vi "myRIO_BRig_RT_dataMTrig_main.vi"(0 "input_dataMTrig":u16[](array[numeric]), 2 "input_Solenoid_trig_L":bool, 3 "input_Solenoid_trig_R":bool, 4 "input_Audio_trig_L":bool, 5 "input_Audio_trig_R":bool, 7 "input_Laser_trig":bool) -> (13 "output_Laser":bool, 14 "output_dataMTrig":u16[](array[numeric]), 16 "output_Solenoid_L":bool, 17 "output_Solenoid_R":bool, 18 "output_Audio_L":bool, 19 "output_Audio_R":bool)   [LabVIEW 2014]
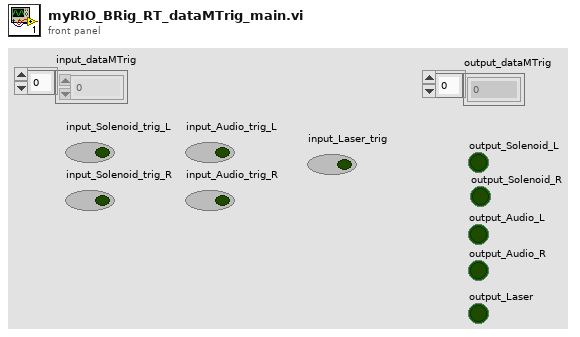
[diagram p1: front panel]
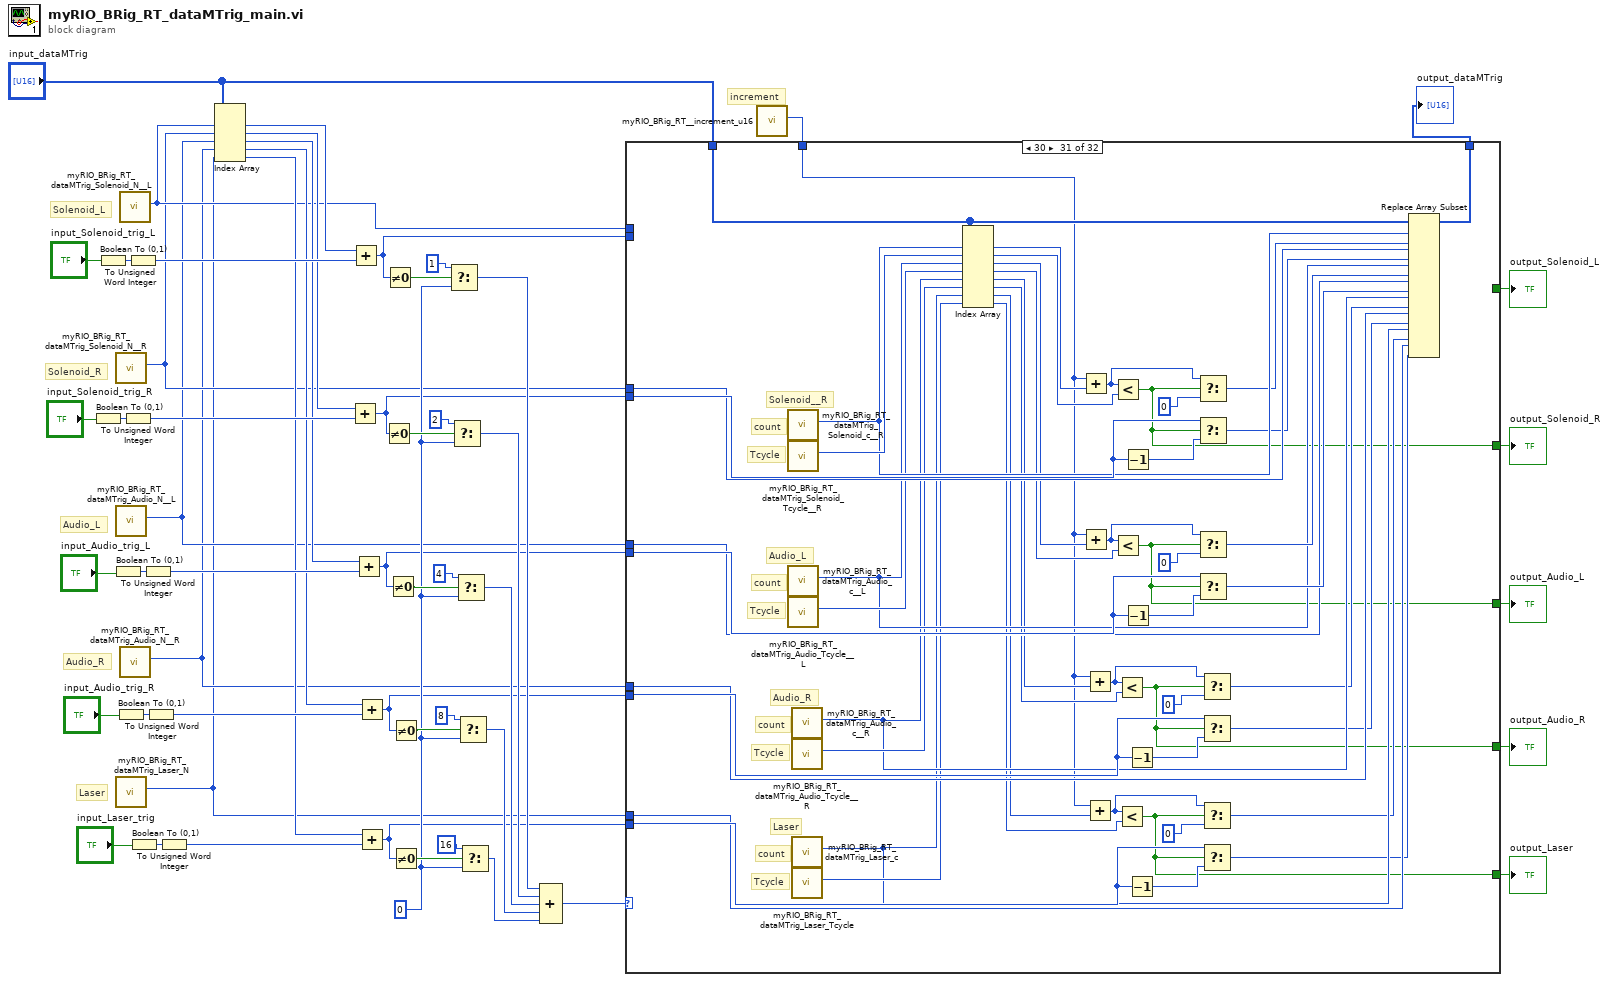
[diagram p0: block diagram]
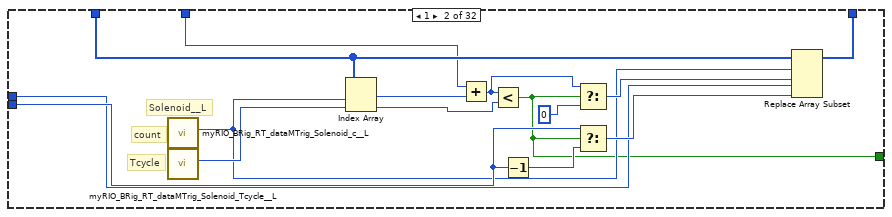
[diagram p3: hidden frame]
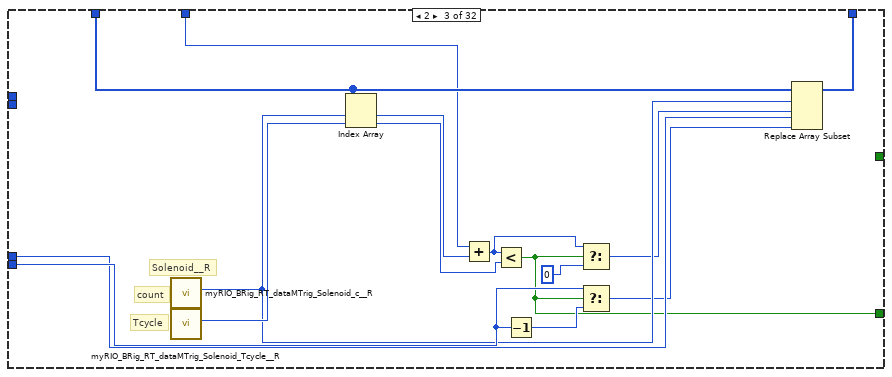
[diagram p4: hidden frame]
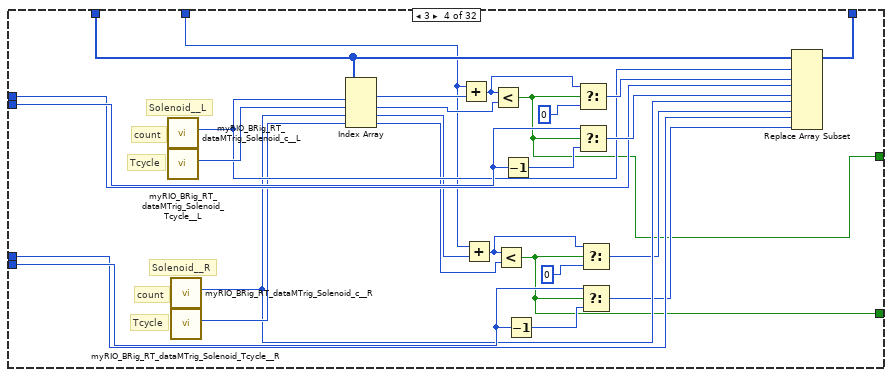
[diagram p5: hidden frame]
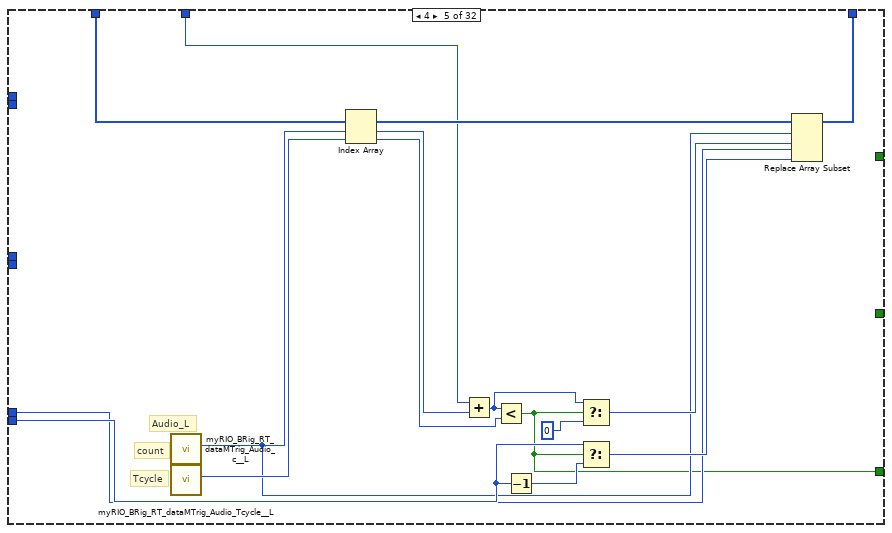
[diagram p6: hidden frame]
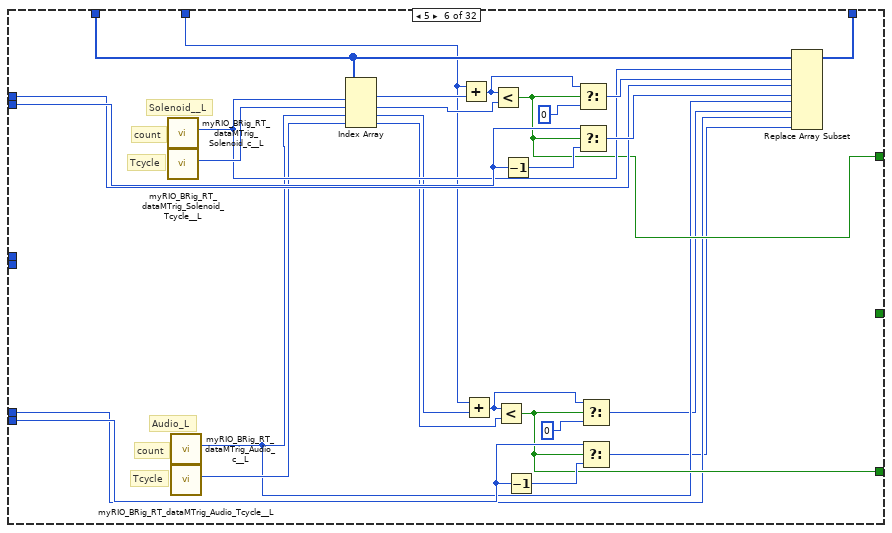
[diagram p7: hidden frame]
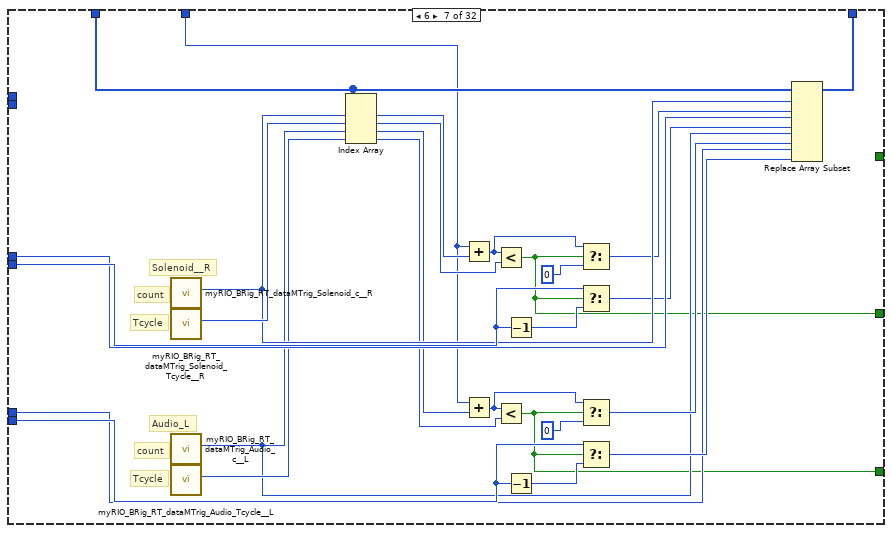
[diagram p8: hidden frame]
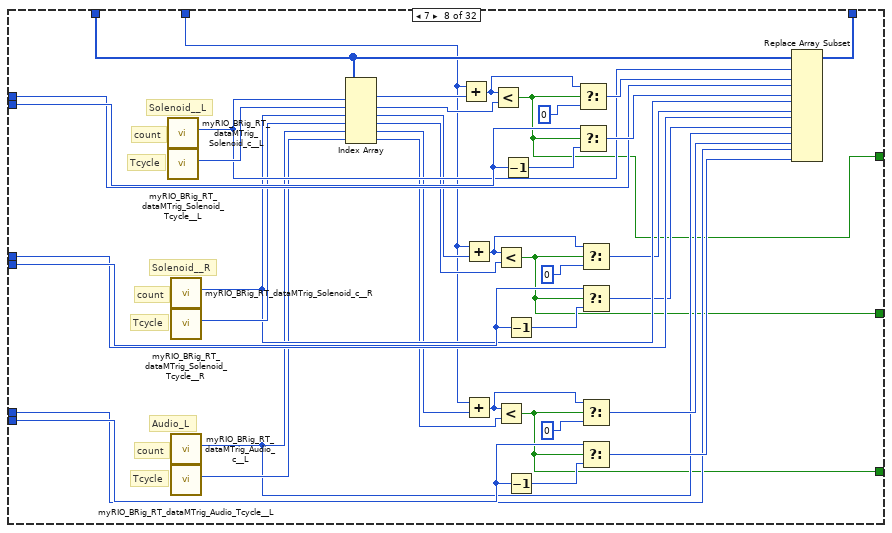
[diagram p9: hidden frame]
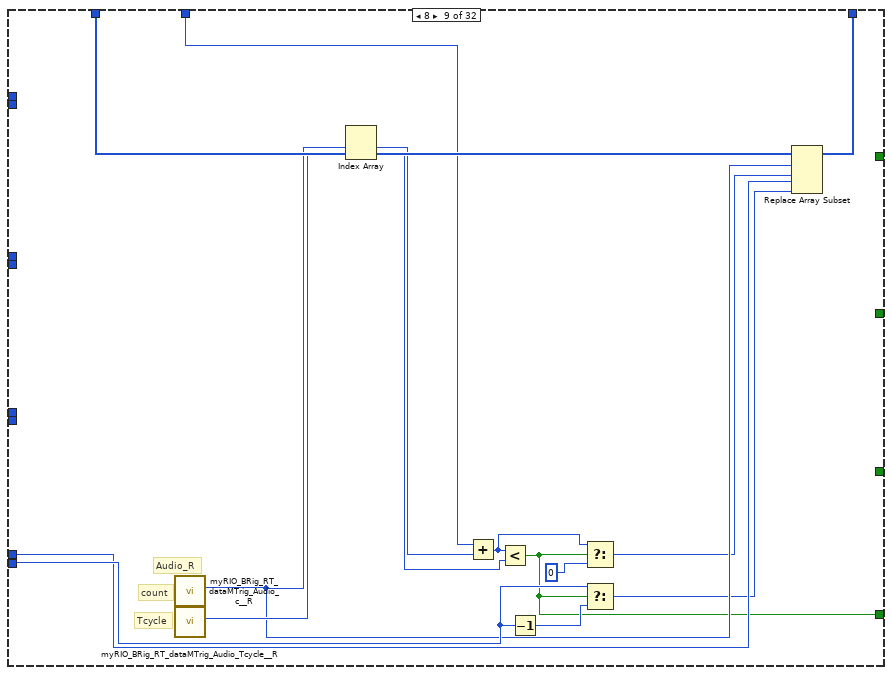
[diagram p10: hidden frame]
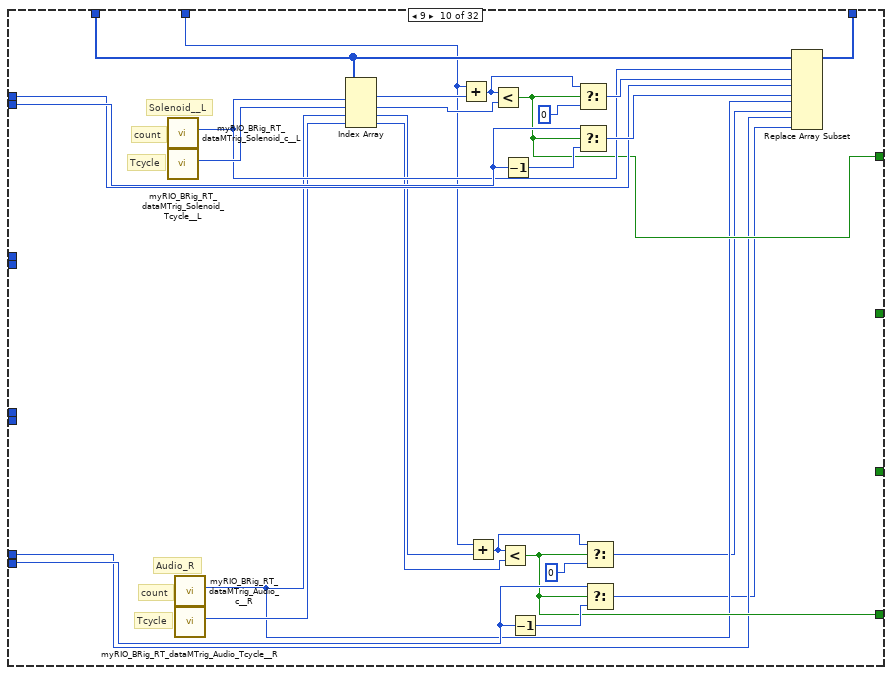
[diagram p11: hidden frame]
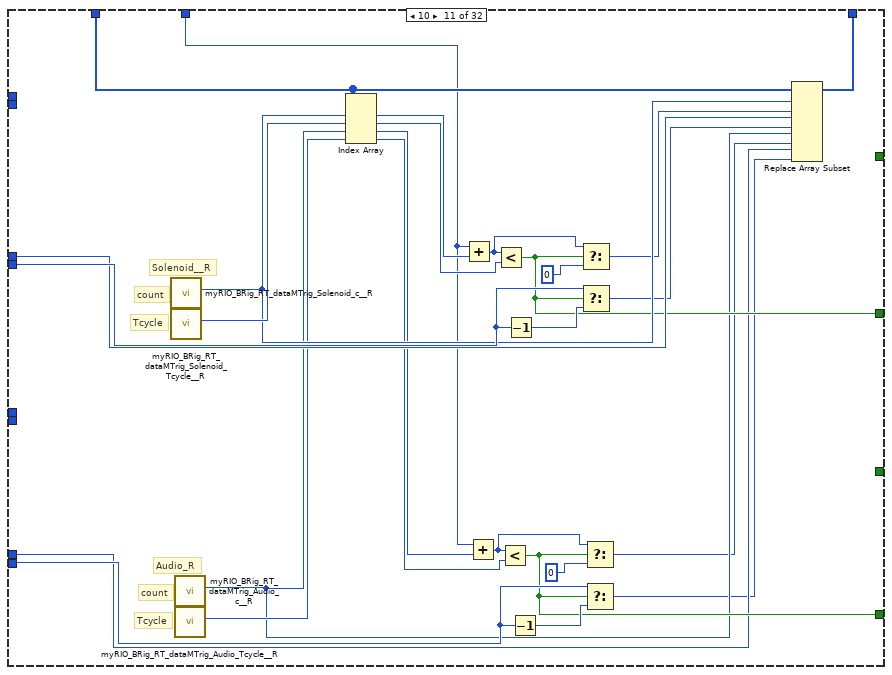
[diagram p12: hidden frame]
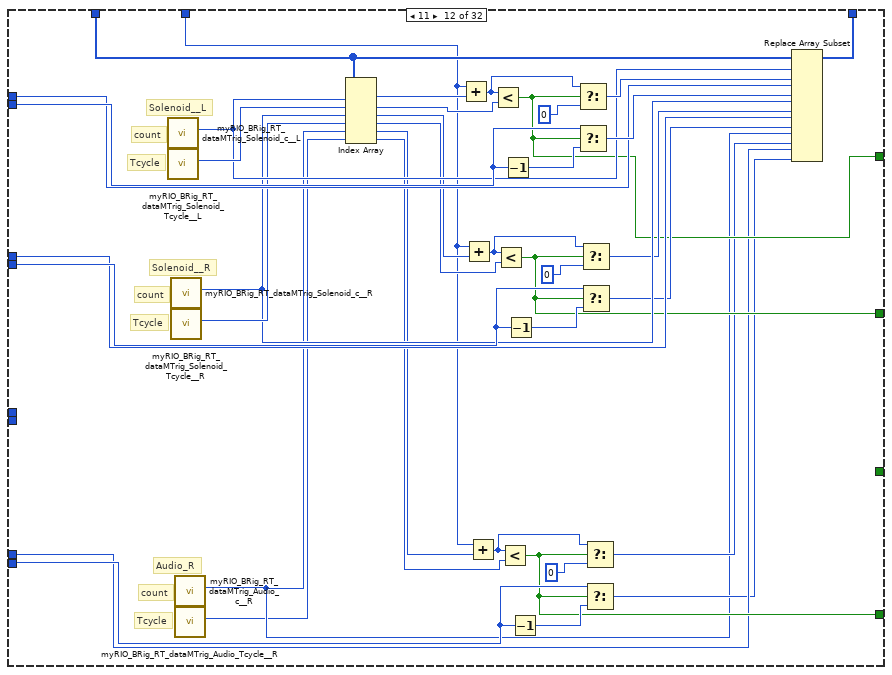
[diagram p13: hidden frame]
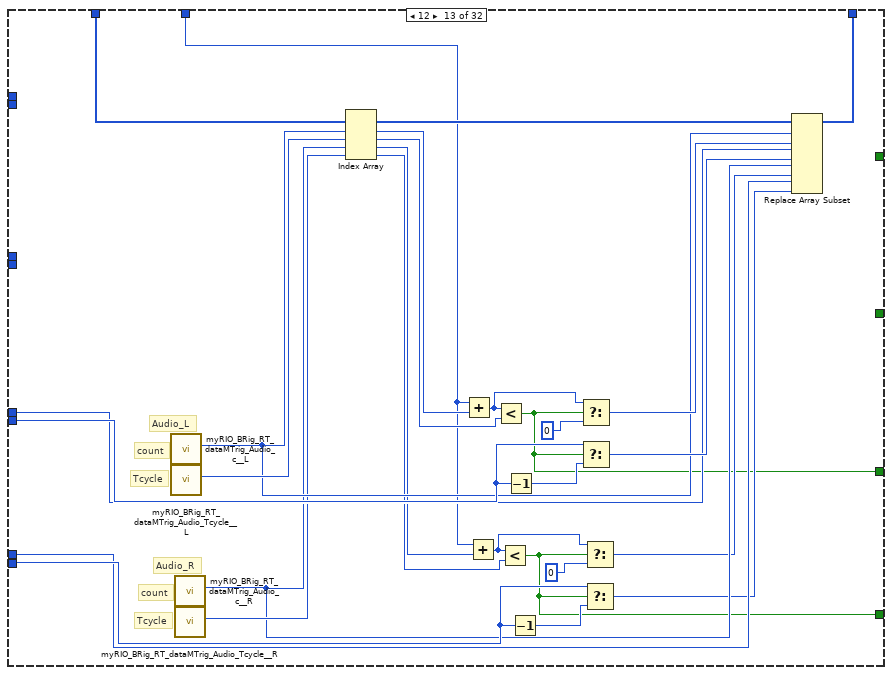
[diagram p14: hidden frame]
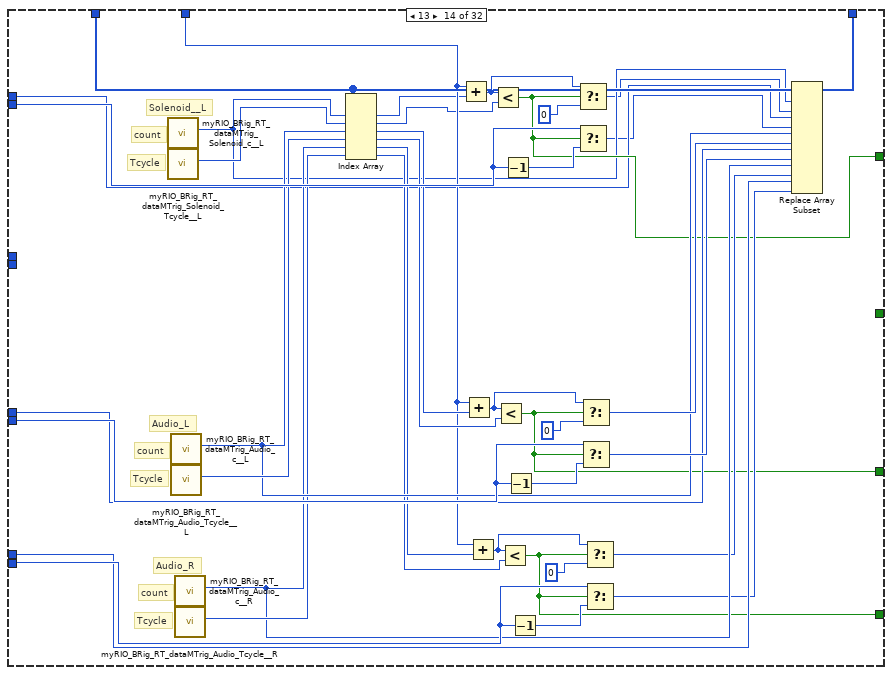
[diagram p15: hidden frame]
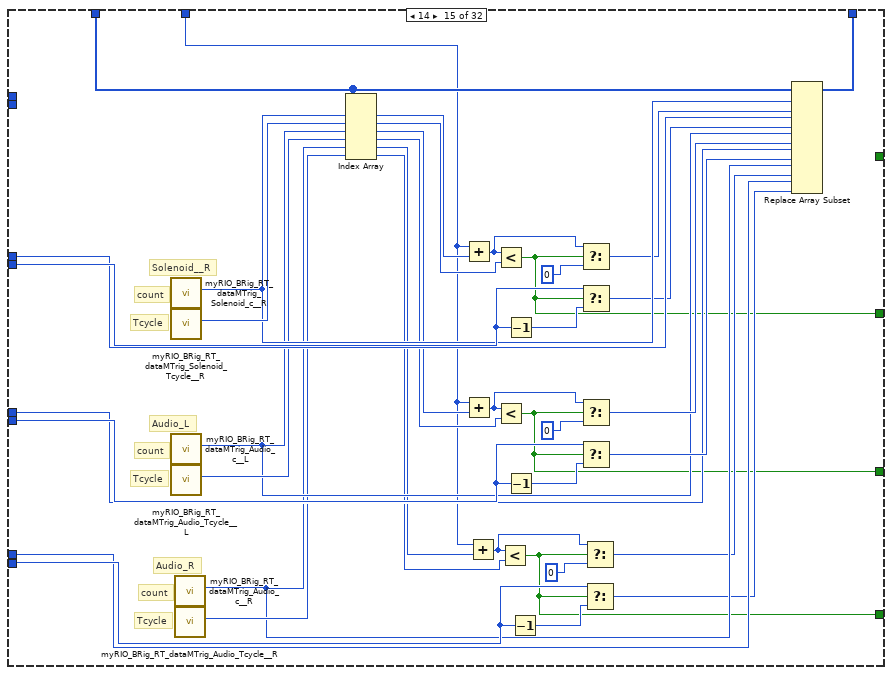
[diagram p16: hidden frame]
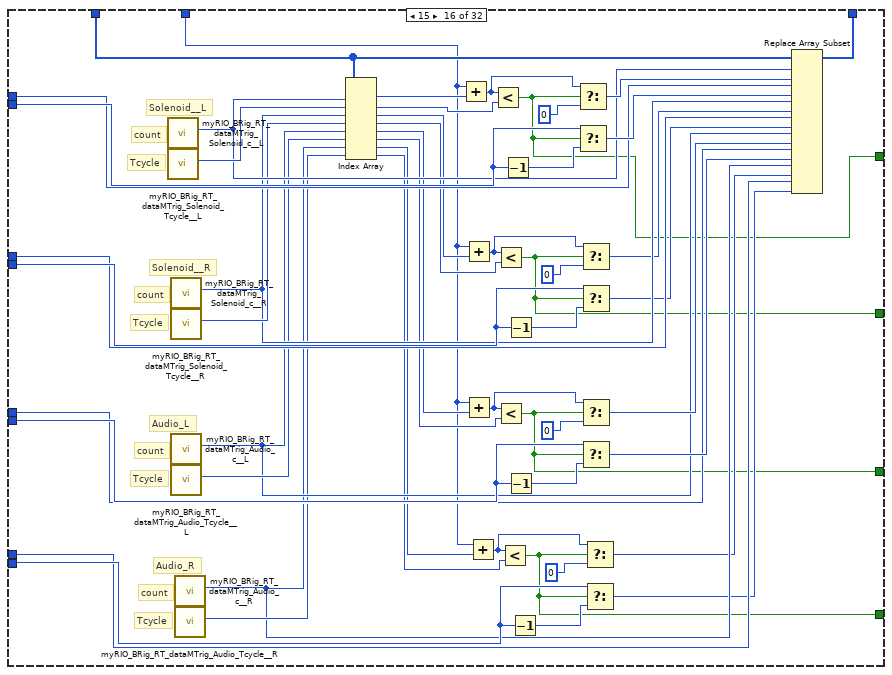
[diagram p17: hidden frame]
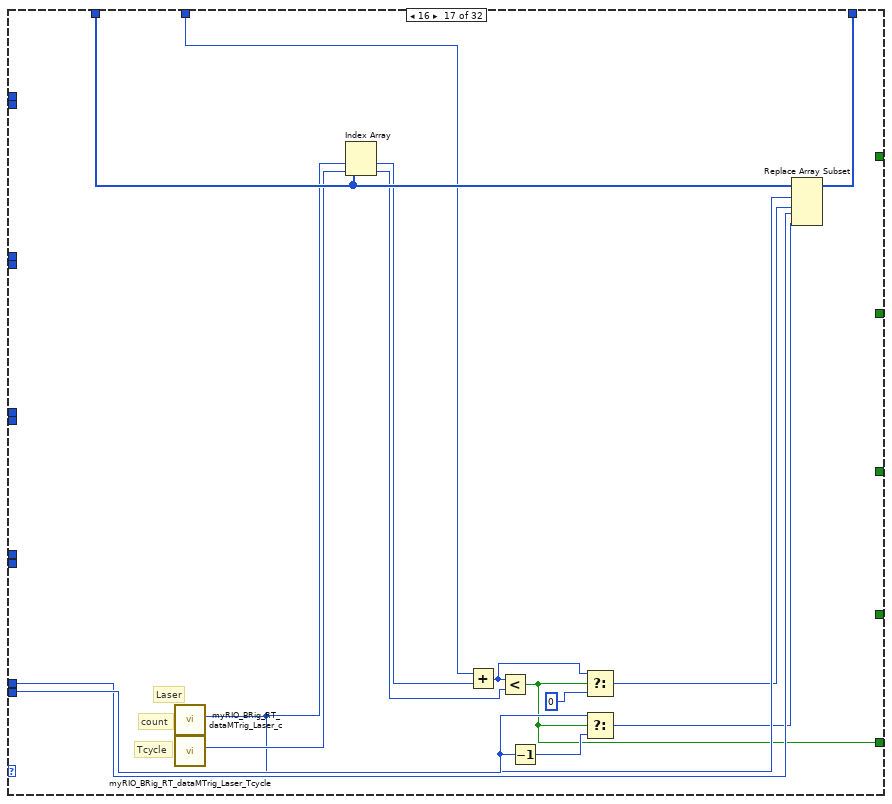
[diagram p18: hidden frame]
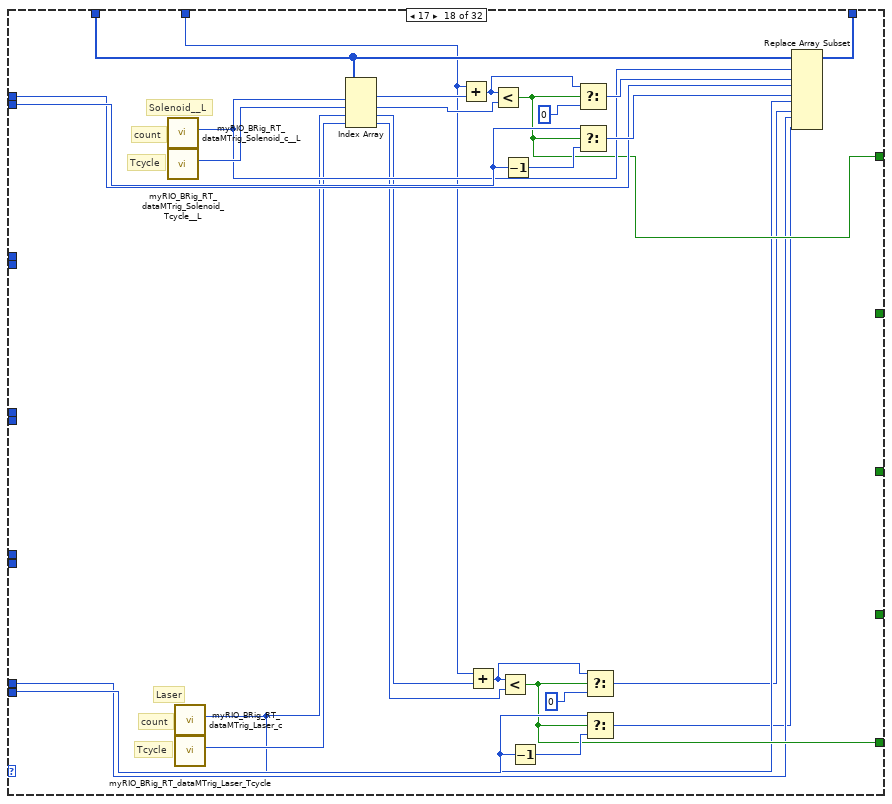
[diagram p19: hidden frame]
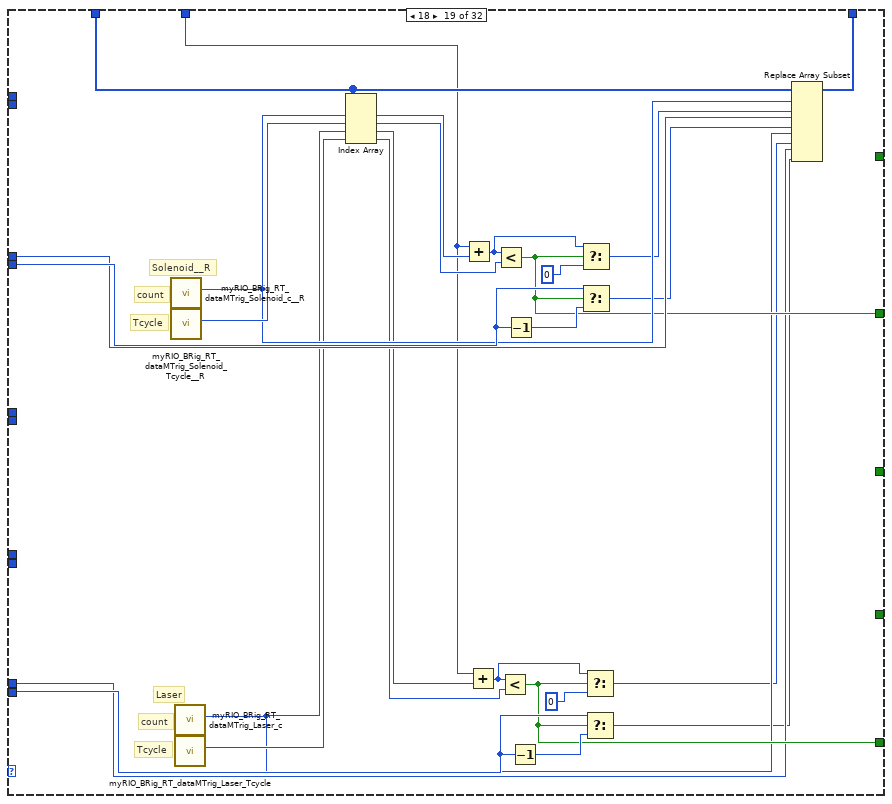
[diagram p20: hidden frame]
diagram:
  w25 = u8 0
  # "increment"
  # "Laser"
  # "Audio_R"
  # "Audio_L"
  # "Solenoid_R"
  # "Solenoid_L"
  n1 = Boolean To (0,1)(Boolean="input_Solenoid_trig_R") -> (0, 1=w53:i16)
  n2 = Boolean To (0,1)(Boolean="input_Solenoid_trig_L") -> (0, 1=w55:i16)
  n3 = Boolean To (0,1)(Boolean="input_Audio_trig_L") -> (0, 1=w51:i16)
  n4 = call "myRIO_BRig_RT_dataMTrig_Solenoid_N__R.vi"() -> ("output_Solenoid_N__R"=w10:i32)  [unwired: 11 in]
  n5 = call "myRIO_BRig_RT_dataMTrig_Audio_N__L.vi"() -> ("output_Audio_N__L"=w8:i32)  [unwired: 11 in]
  n6 = Boolean To (0,1)(Boolean="input_Audio_trig_R") -> (0, 1=w49:i16)
  n7 = call "myRIO_BRig_RT_dataMTrig_Laser_N.vi"() -> ("output_Laser_N"=w6:i32)  [unwired: 11 in]
  n8 = call "myRIO_BRig_RT_dataMTrig_Solenoid_N__L.vi"() -> ("output_Solenoid_N__L"=w11:i32)  [unwired: 11 in]
  n9 = call "myRIO_BRig_RT_dataMTrig_Audio_N__R.vi"() -> ("output_Audio_N__R"=w7:i32)  [unwired: 11 in]
  n10 = To Unsigned Word Integer(number=w53) -> (unsigned 16bit integer=w43:u16)
  n11 = To Unsigned Word Integer(number=w55) -> (unsigned 16bit integer=w45:u16)
  n12 = Boolean To (0,1)(Boolean="input_Laser_trig") -> (0, 1=w47:i16)
  n13 = To Unsigned Word Integer(number=w51) -> (unsigned 16bit integer=w41:u16)
  n14 = To Unsigned Word Integer(number=w49) -> (unsigned 16bit integer=w39:u16)
  n15 = To Unsigned Word Integer(number=w47) -> (unsigned 16bit integer=w37:u16)
  n16 = Index Array(array="input_dataMTrig", index #1=w11, index #2=w10, index #3=w8, index #4=w7, index #5=w6) -> (element #1=w44:u16, element #2=w42:u16, element #3=w40:u16, element #4=w38:u16, element #5=w36:u16)
  n17 = Add(x=w42, y=w43) -> (x+y=w16:u16)
  n18 = Add(x=w44, y=w45) -> (x+y=w18:u16)
  n19 = Add(x=w40, y=w41) -> (x+y=w15:u16)
  n20 = Add(x=w38, y=w39) -> (x+y=w14:u16)
  n21 = Add(x=w36, y=w37) -> (x+y=w13:u16)
  n22 = Not Equal To 0?(x=w16) -> (x != 0?=w26:bool)
  n23 = Not Equal To 0?(x=w18) -> (x != 0?=w35:bool)
  n24 = Not Equal To 0?(x=w15) -> (x != 0?=w27:bool)
  n25 = Not Equal To 0?(x=w14) -> (x != 0?=w28:bool)
  n26 = Not Equal To 0?(x=w13) -> (x != 0?=w29:bool)
  n27 = Select(t=u8 1, s=w35, f=w25) -> (s? t:f=w20:u8)
  n28 = Select(t=u8 2, s=w26, f=w25) -> (s? t:f=w21:u8)
  n29 = Select(t=u8 4, s=w27, f=w25) -> (s? t:f=w22:u8)
  n30 = Select(t=u8 8, s=w28, f=w25) -> (s? t:f=w23:u8)
  n31 = Select(t=u8 16, s=w29, f=w25) -> (s? t:f=w24:u8)
  n32 = Compound Arithmetic op=ADD(w20, w21, w22, w23, w24) -> (w19:u8)
  n33 = call "myRIO_BRig_RT__increment_u16.vi"() -> ("output_increment__u16"=w12:u16)  [unwired: 11 in]
  n34 = case shown="30" w19 {
    tunnel: w18 -> [_ w62 _ w104 _ w146 _ w212 _ w254 _ w320 _ w391 _ w476 _ w518 _ w584 _ w650 _ w740 _ w811 _ w896 _ w991 _ w1100]
    tunnel: "input_dataMTrig" -> [w56 w65 w86 w107 w128 w149 w182 w215 w236 w257 w290 w323 w356 w392 w434 w479 w500 w521 w554 w587 w620 w653 w698 w743 w776 w812 w854 w899 w944 w992 w1046 w1103]
    tunnel: w16 -> [_ _ w82 w98 _ _ w178 w206 _ _ w286 w314 _ _ w430 w470 _ _ w550 w578 _ _ w694 w734 _ _ w850 w890 _ _ w1042 w1094]
    tunnel: w15 -> [_ _ _ _ w123 w139 w166 w194 _ _ _ _ w351 w386 w418 w458 _ _ _ _ w615 w643 w682 w722 _ _ _ _ w939 w986 w1030 w1082]
    tunnel: w14 -> [_ _ _ _ _ _ _ _ w231 w247 w274 w302 w340 w375 w407 w447 _ _ _ _ _ _ _ _ w771 w806 w845 w878 w928 w975 w1019 w1071]
    tunnel: w13 -> [_ _ _ _ _ _ _ _ _ _ _ _ _ _ _ _ w495 w511 w538 w566 w604 w639 w671 w711 w760 w795 w834 w874 w917 w964 w1008 w1060]
    tunnel: w12 -> [_ w58 w73 w89 w115 w138 w158 w186 w223 w246 w273 w301 w332 w367 w399 w439 w494 w510 w537 w565 w603 w638 w670 w710 w759 w794 w833 w873 w916 w963 w1007 w1059]
    tunnel: w11 -> [_ w61 _ w103 _ w145 _ w211 _ w253 _ w319 _ w358 _ w475 _ w517 _ w583 _ w649 _ w739 _ w778 _ w895 _ w946 _ w1099]
    tunnel: w10 -> [_ _ w76 w92 _ _ w172 w200 _ _ w280 w308 _ _ w424 w464 _ _ w544 w572 _ _ w688 w728 _ _ w821 w884 _ _ w1036 w1088]
    tunnel: [w56 w59 w74 w90 w127 w143 w170 w198 w235 w251 w278 w306 w355 w390 w422 w462 w499 w515 w542 w570 w619 w647 w686 w726 w775 w810 w849 w882 w943 w990 w1034 w1086] -> w9
    tunnel: w8 -> [_ _ _ _ w117 w130 w160 w188 _ _ _ _ w345 w380 w412 w452 _ _ _ _ w609 w626 w676 w716 _ _ _ _ w933 w980 w1024 w1076]
    tunnel: w7 -> [_ _ _ _ _ _ _ _ w226 w238 w265 w296 w335 w370 w402 w442 _ _ _ _ _ _ _ _ w766 w801 w840 w860 w923 w970 w1014 w1066]
    tunnel: w6 -> [_ _ _ _ _ _ _ _ _ _ _ _ _ _ _ _ w489 w502 w529 w556 w595 w622 w661 w700 w754 w789 w828 w856 w911 w958 w1002 w1054]
    tunnel: [_ _ _ _ _ _ _ _ _ _ _ _ _ _ _ _ w486 w509 w536 w564 w602 w637 w669 w709 w751 w786 w825 w872 w908 w955 w999 w1051] -> w1
    tunnel: [_ _ _ _ _ _ _ _ w222 w245 w272 w300 w331 w366 w398 w438 _ _ _ _ _ _ _ _ w750 w785 w824 w871 w907 w954 w998 w1050] -> w2
    tunnel: [_ _ _ _ w114 w137 w157 w185 _ _ _ _ w330 w365 w397 w437 _ _ _ _ w601 w636 w668 w708 _ _ _ _ w906 w953 w997 w1049] -> w3
    tunnel: [_ _ w72 w88 _ _ w156 w184 _ _ w271 w299 _ _ w396 w436 _ _ w535 w563 _ _ w667 w707 _ _ w823 w870 _ _ w996 w1048] -> w4
    tunnel: [_ w57 _ w87 _ w136 _ w183 _ w244 _ w298 _ w364 _ w435 _ w508 _ w562 _ w635 _ w706 _ w784 _ w869 _ w952 _ w1047] -> w5
    frame 0, Default {
    }
    frame 1 {
      # "Solenoid__L"
      # "Tcycle"
      # "count"
      n35 = call "myRIO_BRig_RT_dataMTrig_Solenoid_c__L.vi"() -> ("output_Solenoid_c__L"=w60:i32)  [unwired: 11 in]
      n36 = call "myRIO_BRig_RT_dataMTrig_Solenoid_Tcycle__L.vi"() -> ("output_Solenoid_Tcycle__L"=w71:i32)  [unwired: 11 in]
      n37 = Index Array(array=w65, index #1=w60, index #2=w71) -> (element #1=w70:u16, element #2=w69:u16)
      n38 = Add(x=w58, y=w70) -> (x+y=w67:u16)
      n39 = Less?(x=w67, y=w69) -> (x < y?=w57:bool)
      n40 = Decrement(x=w62) -> (x-1=w68:u16)
      n41 = Select(t=w67, s=w57, f=u16 0) -> (s? t:f=w63:u16)
      n42 = Select(t=w62, s=w57, f=w68) -> (s? t:f=w64:u16)
      n43 = Replace Array Subset(array=w65, new element #1=w63, index #1=w60, new element #2=w64, index #2=w61) -> (w59:u16[])
    }
    frame 2 {
      # "Solenoid__R"
      # "Tcycle"
      # "count"
      n44 = call "myRIO_BRig_RT_dataMTrig_Solenoid_c__R.vi"() -> ("output_Solenoid_c__R"=w78:i32)  [unwired: 11 in]
      n45 = call "myRIO_BRig_RT_dataMTrig_Solenoid_Tcycle__R.vi"() -> ("output_Solenoid_Tcycle__R"=w81:i32)  [unwired: 11 in]
      n46 = Index Array(array=w86, index #1=w78, index #2=w81) -> (element #1=w80:u16, element #2=w79:u16)
      n47 = Add(x=w73, y=w80) -> (x+y=w84:u16)
      n48 = Less?(x=w84, y=w79) -> (x < y?=w72:bool)
      n49 = Decrement(x=w82) -> (x-1=w85:u16)
      n50 = Select(t=w84, s=w72, f=u16 0) -> (s? t:f=w77:u16)
      n51 = Select(t=w82, s=w72, f=w85) -> (s? t:f=w75:u16)
      n52 = Replace Array Subset(array=w86, new element #1=w77, index #1=w78, new element #2=w75, index #2=w76) -> (w74:u16[])
    }
    frame 3 {
      # "Solenoid__R"
      # "Tcycle"
      # "count"
      # "Solenoid__L"
      # "Tcycle"
      # "count"
      n53 = call "myRIO_BRig_RT_dataMTrig_Solenoid_c__L.vi"() -> ("output_Solenoid_c__L"=w102:i32)  [unwired: 11 in]
      n54 = call "myRIO_BRig_RT_dataMTrig_Solenoid_Tcycle__L.vi"() -> ("output_Solenoid_Tcycle__L"=w113:i32)  [unwired: 11 in]
      n55 = call "myRIO_BRig_RT_dataMTrig_Solenoid_c__R.vi"() -> ("output_Solenoid_c__R"=w94:i32)  [unwired: 11 in]
      n56 = call "myRIO_BRig_RT_dataMTrig_Solenoid_Tcycle__R.vi"() -> ("output_Solenoid_Tcycle__R"=w97:i32)  [unwired: 11 in]
      n57 = Index Array(array=w107, index #1=w102, index #2=w113, index #3=w94, index #4=w97) -> (element #1=w112:u16, element #2=w111:u16, element #3=w96:u16, element #4=w95:u16)
      n58 = Add(x=w89, y=w112) -> (x+y=w109:u16)
      n59 = Add(x=w89, y=w96) -> (x+y=w100:u16)
      n60 = Less?(x=w109, y=w111) -> (x < y?=w87:bool)
      n61 = Less?(x=w100, y=w95) -> (x < y?=w88:bool)
      n62 = Decrement(x=w104) -> (x-1=w110:u16)
      n63 = Decrement(x=w98) -> (x-1=w101:u16)
      n64 = Select(t=w109, s=w87, f=u16 0) -> (s? t:f=w105:u16)
      n65 = Select(t=w104, s=w87, f=w110) -> (s? t:f=w106:u16)
      n66 = Select(t=w100, s=w88, f=u16 0) -> (s? t:f=w93:u16)
      n67 = Select(t=w98, s=w88, f=w101) -> (s? t:f=w91:u16)
      n68 = Replace Array Subset(array=w107, new element #1=w105, index #1=w102, new element #2=w106, index #2=w103, new element #3=w93, index #3=w94, new element #4=w91, index #4=w92) -> (w90:u16[])
    }
    frame 4 {
      # "Audio_L"
      # "Tcycle"
      # "count"
      n69 = call "myRIO_BRig_RT_dataMTrig_Audio_c__L.vi"() -> ("output_Audio_c__L"=w116:i32)  [unwired: 11 in]
      n70 = call "myRIO_BRig_RT_dataMTrig_Audio_Tcycle__L.vi"() -> ("output_Audio_Tcycle__L"=w122:i32)  [unwired: 11 in]
      n71 = Index Array(array=w128, index #1=w116, index #2=w122) -> (element #1=w121:u16, element #2=w120:u16)
      n72 = Add(x=w115, y=w121) -> (x+y=w125:u16)
      n73 = Less?(x=w125, y=w120) -> (x < y?=w114:bool)
      n74 = Decrement(x=w123) -> (x-1=w126:u16)
      n75 = Select(t=w125, s=w114, f=u16 0) -> (s? t:f=w119:u16)
      n76 = Select(t=w123, s=w114, f=w126) -> (s? t:f=w118:u16)
      n77 = Replace Array Subset(array=w128, new element #1=w119, index #1=w116, new element #2=w118, index #2=w117) -> (w127:u16[])
    }
    frame 5 {
      # "Audio_L"
      # "Tcycle"
      # "count"
      # "Solenoid__L"
      # "Tcycle"
      # "count"
      n78 = call "myRIO_BRig_RT_dataMTrig_Solenoid_c__L.vi"() -> ("output_Solenoid_c__L"=w144:i32)  [unwired: 11 in]
      n79 = call "myRIO_BRig_RT_dataMTrig_Solenoid_Tcycle__L.vi"() -> ("output_Solenoid_Tcycle__L"=w155:i32)  [unwired: 11 in]
      n80 = call "myRIO_BRig_RT_dataMTrig_Audio_c__L.vi"() -> ("output_Audio_c__L"=w132:i32)  [unwired: 11 in]
      n81 = call "myRIO_BRig_RT_dataMTrig_Audio_Tcycle__L.vi"() -> ("output_Audio_Tcycle__L"=w135:i32)  [unwired: 11 in]
      n82 = Index Array(array=w149, index #1=w144, index #2=w155, index #3=w132, index #4=w135) -> (element #1=w154:u16, element #2=w153:u16, element #3=w134:u16, element #4=w133:u16)
      n83 = Add(x=w138, y=w154) -> (x+y=w151:u16)
      n84 = Add(x=w138, y=w134) -> (x+y=w141:u16)
      n85 = Less?(x=w151, y=w153) -> (x < y?=w136:bool)
      n86 = Less?(x=w141, y=w133) -> (x < y?=w137:bool)
      n87 = Decrement(x=w146) -> (x-1=w152:u16)
      n88 = Decrement(x=w139) -> (x-1=w142:u16)
      n89 = Select(t=w151, s=w136, f=u16 0) -> (s? t:f=w147:u16)
      n90 = Select(t=w146, s=w136, f=w152) -> (s? t:f=w148:u16)
      n91 = Select(t=w141, s=w137, f=u16 0) -> (s? t:f=w131:u16)
      n92 = Select(t=w139, s=w137, f=w142) -> (s? t:f=w129:u16)
      n93 = Replace Array Subset(array=w149, new element #1=w147, index #1=w144, new element #2=w148, index #2=w145, new element #3=w131, index #3=w132, new element #4=w129, index #4=w130) -> (w143:u16[])
    }
    frame 6 {
      # "Audio_L"
      # "Tcycle"
      # "count"
      # "Solenoid__R"
      # "Tcycle"
      # "count"
      n94 = call "myRIO_BRig_RT_dataMTrig_Solenoid_c__R.vi"() -> ("output_Solenoid_c__R"=w174:i32)  [unwired: 11 in]
      n95 = call "myRIO_BRig_RT_dataMTrig_Solenoid_Tcycle__R.vi"() -> ("output_Solenoid_Tcycle__R"=w177:i32)  [unwired: 11 in]
      n96 = call "myRIO_BRig_RT_dataMTrig_Audio_c__L.vi"() -> ("output_Audio_c__L"=w159:i32)  [unwired: 11 in]
      n97 = call "myRIO_BRig_RT_dataMTrig_Audio_Tcycle__L.vi"() -> ("output_Audio_Tcycle__L"=w165:i32)  [unwired: 11 in]
      n98 = Index Array(array=w182, index #1=w174, index #2=w177, index #3=w159, index #4=w165) -> (element #1=w176:u16, element #2=w175:u16, element #3=w164:u16, element #4=w163:u16)
      n99 = Add(x=w158, y=w176) -> (x+y=w180:u16)
      n100 = Add(x=w158, y=w164) -> (x+y=w168:u16)
      n101 = Less?(x=w180, y=w175) -> (x < y?=w156:bool)
      n102 = Less?(x=w168, y=w163) -> (x < y?=w157:bool)
      n103 = Decrement(x=w178) -> (x-1=w181:u16)
      n104 = Decrement(x=w166) -> (x-1=w169:u16)
      n105 = Select(t=w180, s=w156, f=u16 0) -> (s? t:f=w173:u16)
      n106 = Select(t=w178, s=w156, f=w181) -> (s? t:f=w171:u16)
      n107 = Select(t=w168, s=w157, f=u16 0) -> (s? t:f=w162:u16)
      n108 = Select(t=w166, s=w157, f=w169) -> (s? t:f=w161:u16)
      n109 = Replace Array Subset(array=w182, new element #1=w173, index #1=w174, new element #2=w171, index #2=w172, new element #3=w162, index #3=w159, new element #4=w161, index #4=w160) -> (w170:u16[])
    }
    frame 7 {
      # "Audio_L"
      # "Tcycle"
      # "count"
      # "Solenoid__R"
      # "Tcycle"
      # "count"
      # "Solenoid__L"
      # "Tcycle"
      # "count"
      n110 = call "myRIO_BRig_RT_dataMTrig_Solenoid_c__L.vi"() -> ("output_Solenoid_c__L"=w210:i32)  [unwired: 11 in]
      n111 = call "myRIO_BRig_RT_dataMTrig_Solenoid_Tcycle__L.vi"() -> ("output_Solenoid_Tcycle__L"=w221:i32)  [unwired: 11 in]
      n112 = call "myRIO_BRig_RT_dataMTrig_Solenoid_c__R.vi"() -> ("output_Solenoid_c__R"=w202:i32)  [unwired: 11 in]
      n113 = call "myRIO_BRig_RT_dataMTrig_Solenoid_Tcycle__R.vi"() -> ("output_Solenoid_Tcycle__R"=w205:i32)  [unwired: 11 in]
      n114 = call "myRIO_BRig_RT_dataMTrig_Audio_c__L.vi"() -> ("output_Audio_c__L"=w187:i32)  [unwired: 11 in]
      n115 = call "myRIO_BRig_RT_dataMTrig_Audio_Tcycle__L.vi"() -> ("output_Audio_Tcycle__L"=w193:i32)  [unwired: 11 in]
      n116 = Index Array(array=w215, index #1=w210, index #2=w221, index #3=w202, index #4=w205, index #5=w187, index #6=w193) -> (element #1=w220:u16, element #2=w219:u16, element #3=w204:u16, element #4=w203:u16, element #5=w192:u16, element #6=w191:u16)
      n117 = Add(x=w186, y=w220) -> (x+y=w217:u16)
      n118 = Add(x=w186, y=w204) -> (x+y=w208:u16)
      n119 = Add(x=w186, y=w192) -> (x+y=w196:u16)
      n120 = Less?(x=w217, y=w219) -> (x < y?=w183:bool)
      n121 = Less?(x=w208, y=w203) -> (x < y?=w184:bool)
      n122 = Less?(x=w196, y=w191) -> (x < y?=w185:bool)
      n123 = Decrement(x=w212) -> (x-1=w218:u16)
      n124 = Decrement(x=w206) -> (x-1=w209:u16)
      n125 = Decrement(x=w194) -> (x-1=w197:u16)
      n126 = Select(t=w217, s=w183, f=u16 0) -> (s? t:f=w213:u16)
      n127 = Select(t=w212, s=w183, f=w218) -> (s? t:f=w214:u16)
      n128 = Select(t=w208, s=w184, f=u16 0) -> (s? t:f=w201:u16)
      n129 = Select(t=w206, s=w184, f=w209) -> (s? t:f=w199:u16)
      n130 = Select(t=w196, s=w185, f=u16 0) -> (s? t:f=w190:u16)
      n131 = Select(t=w194, s=w185, f=w197) -> (s? t:f=w189:u16)
      n132 = Replace Array Subset(array=w215, new element #1=w213, index #1=w210, new element #2=w214, index #2=w211, new element #3=w201, index #3=w202, new element #4=w199, index #4=w200, new element #5=w190, index #5=w187, new element #6=w189, index #6=w188) -> (w198:u16[])
    }
    frame 8 {
      # "Audio_R"
      # "Tcycle"
      # "count"
      n133 = call "myRIO_BRig_RT_dataMTrig_Audio_c__R.vi"() -> ("output_Audio_c__R"=w227:i32)  [unwired: 11 in]
      n134 = call "myRIO_BRig_RT_dataMTrig_Audio_Tcycle__R.vi"() -> ("output_Audio_Tcycle__R"=w228:i32)  [unwired: 11 in]
      n135 = Index Array(array=w236, index #1=w227, index #2=w228) -> (element #1=w230:u16, element #2=w229:u16)
      n136 = Add(x=w223, y=w230) -> (x+y=w233:u16)
      n137 = Less?(x=w233, y=w229) -> (x < y?=w222:bool)
      n138 = Decrement(x=w231) -> (x-1=w234:u16)
      n139 = Select(t=w233, s=w222, f=u16 0) -> (s? t:f=w225:u16)
      n140 = Select(t=w231, s=w222, f=w234) -> (s? t:f=w224:u16)
      n141 = Replace Array Subset(array=w236, new element #1=w225, index #1=w227, new element #2=w224, index #2=w226) -> (w235:u16[])
    }
    frame 9 {
      # "Audio_R"
      # "Tcycle"
      # "count"
      # "Solenoid__L"
      # "Tcycle"
      # "count"
      n142 = call "myRIO_BRig_RT_dataMTrig_Solenoid_c__L.vi"() -> ("output_Solenoid_c__L"=w252:i32)  [unwired: 11 in]
      n143 = call "myRIO_BRig_RT_dataMTrig_Solenoid_Tcycle__L.vi"() -> ("output_Solenoid_Tcycle__L"=w263:i32)  [unwired: 11 in]
      n144 = call "myRIO_BRig_RT_dataMTrig_Audio_c__R.vi"() -> ("output_Audio_c__R"=w240:i32)  [unwired: 11 in]
      n145 = call "myRIO_BRig_RT_dataMTrig_Audio_Tcycle__R.vi"() -> ("output_Audio_Tcycle__R"=w243:i32)  [unwired: 11 in]
      n146 = Index Array(array=w257, index #1=w252, index #2=w263, index #3=w240, index #4=w243) -> (element #1=w262:u16, element #2=w261:u16, element #3=w242:u16, element #4=w241:u16)
      n147 = Add(x=w246, y=w262) -> (x+y=w259:u16)
      n148 = Add(x=w246, y=w242) -> (x+y=w249:u16)
      n149 = Less?(x=w259, y=w261) -> (x < y?=w244:bool)
      n150 = Less?(x=w249, y=w241) -> (x < y?=w245:bool)
      n151 = Decrement(x=w254) -> (x-1=w260:u16)
      n152 = Decrement(x=w247) -> (x-1=w250:u16)
      n153 = Select(t=w259, s=w244, f=u16 0) -> (s? t:f=w255:u16)
      n154 = Select(t=w254, s=w244, f=w260) -> (s? t:f=w256:u16)
      n155 = Select(t=w249, s=w245, f=u16 0) -> (s? t:f=w239:u16)
      n156 = Select(t=w247, s=w245, f=w250) -> (s? t:f=w237:u16)
      n157 = Replace Array Subset(array=w257, new element #1=w255, index #1=w252, new element #2=w256, index #2=w253, new element #3=w239, index #3=w240, new element #4=w237, index #4=w238) -> (w251:u16[])
    }
    frame 10 {
      # "Audio_R"
      # "Tcycle"
      # "count"
      # "Solenoid__R"
      # "Tcycle"
      # "count"
      n158 = call "myRIO_BRig_RT_dataMTrig_Solenoid_c__R.vi"() -> ("output_Solenoid_c__R"=w282:i32)  [unwired: 11 in]
      n159 = call "myRIO_BRig_RT_dataMTrig_Solenoid_Tcycle__R.vi"() -> ("output_Solenoid_Tcycle__R"=w285:i32)  [unwired: 11 in]
      n160 = call "myRIO_BRig_RT_dataMTrig_Audio_c__R.vi"() -> ("output_Audio_c__R"=w267:i32)  [unwired: 11 in]
      n161 = call "myRIO_BRig_RT_dataMTrig_Audio_Tcycle__R.vi"() -> ("output_Audio_Tcycle__R"=w270:i32)  [unwired: 11 in]
      n162 = Index Array(array=w290, index #1=w282, index #2=w285, index #3=w267, index #4=w270) -> (element #1=w284:u16, element #2=w283:u16, element #3=w269:u16, element #4=w268:u16)
      n163 = Add(x=w273, y=w284) -> (x+y=w288:u16)
      n164 = Add(x=w273, y=w269) -> (x+y=w276:u16)
      n165 = Less?(x=w288, y=w283) -> (x < y?=w271:bool)
      n166 = Less?(x=w276, y=w268) -> (x < y?=w272:bool)
      n167 = Decrement(x=w286) -> (x-1=w289:u16)
      n168 = Decrement(x=w274) -> (x-1=w277:u16)
      n169 = Select(t=w288, s=w271, f=u16 0) -> (s? t:f=w281:u16)
      n170 = Select(t=w286, s=w271, f=w289) -> (s? t:f=w279:u16)
      n171 = Select(t=w276, s=w272, f=u16 0) -> (s? t:f=w266:u16)
      n172 = Select(t=w274, s=w272, f=w277) -> (s? t:f=w264:u16)
      n173 = Replace Array Subset(array=w290, new element #1=w281, index #1=w282, new element #2=w279, index #2=w280, new element #3=w266, index #3=w267, new element #4=w264, index #4=w265) -> (w278:u16[])
    }
    frame 11 {
      # "Audio_R"
      # "Tcycle"
      # "count"
      # "Solenoid__R"
      # "Tcycle"
      # "count"
      # "Solenoid__L"
      # "Tcycle"
      # "count"
      n174 = call "myRIO_BRig_RT_dataMTrig_Solenoid_c__L.vi"() -> ("output_Solenoid_c__L"=w318:i32)  [unwired: 11 in]
      n175 = call "myRIO_BRig_RT_dataMTrig_Solenoid_Tcycle__L.vi"() -> ("output_Solenoid_Tcycle__L"=w329:i32)  [unwired: 11 in]
      n176 = call "myRIO_BRig_RT_dataMTrig_Solenoid_c__R.vi"() -> ("output_Solenoid_c__R"=w310:i32)  [unwired: 11 in]
      n177 = call "myRIO_BRig_RT_dataMTrig_Solenoid_Tcycle__R.vi"() -> ("output_Solenoid_Tcycle__R"=w313:i32)  [unwired: 11 in]
      n178 = call "myRIO_BRig_RT_dataMTrig_Audio_c__R.vi"() -> ("output_Audio_c__R"=w294:i32)  [unwired: 11 in]
      n179 = call "myRIO_BRig_RT_dataMTrig_Audio_Tcycle__R.vi"() -> ("output_Audio_Tcycle__R"=w293:i32)  [unwired: 11 in]
      n180 = Index Array(array=w323, index #1=w318, index #2=w329, index #3=w310, index #4=w313, index #5=w294, index #6=w293) -> (element #1=w328:u16, element #2=w327:u16, element #3=w312:u16, element #4=w311:u16, element #5=w292:u16, element #6=w291:u16)
      n181 = Add(x=w301, y=w328) -> (x+y=w325:u16)
      n182 = Add(x=w301, y=w312) -> (x+y=w316:u16)
      n183 = Add(x=w301, y=w292) -> (x+y=w304:u16)
      n184 = Less?(x=w325, y=w327) -> (x < y?=w298:bool)
      n185 = Less?(x=w316, y=w311) -> (x < y?=w299:bool)
      n186 = Less?(x=w304, y=w291) -> (x < y?=w300:bool)
      n187 = Decrement(x=w320) -> (x-1=w326:u16)
      n188 = Decrement(x=w314) -> (x-1=w317:u16)
      n189 = Decrement(x=w302) -> (x-1=w305:u16)
      n190 = Select(t=w325, s=w298, f=u16 0) -> (s? t:f=w321:u16)
      n191 = Select(t=w320, s=w298, f=w326) -> (s? t:f=w322:u16)
      n192 = Select(t=w316, s=w299, f=u16 0) -> (s? t:f=w309:u16)
      n193 = Select(t=w314, s=w299, f=w317) -> (s? t:f=w307:u16)
      n194 = Select(t=w304, s=w300, f=u16 0) -> (s? t:f=w297:u16)
      n195 = Select(t=w302, s=w300, f=w305) -> (s? t:f=w295:u16)
      n196 = Replace Array Subset(array=w323, new element #1=w321, index #1=w318, new element #2=w322, index #2=w319, new element #3=w309, index #3=w310, new element #4=w307, index #4=w308, new element #5=w297, index #5=w294, new element #6=w295, index #6=w296) -> (w306:u16[])
    }
    frame 12 {
      # "Audio_R"
      # "Tcycle"
      # "count"
      # "Audio_L"
      # "Tcycle"
      # "count"
      n197 = call "myRIO_BRig_RT_dataMTrig_Audio_c__L.vi"() -> ("output_Audio_c__L"=w344:i32)  [unwired: 11 in]
      n198 = call "myRIO_BRig_RT_dataMTrig_Audio_Tcycle__L.vi"() -> ("output_Audio_Tcycle__L"=w350:i32)  [unwired: 11 in]
      n199 = call "myRIO_BRig_RT_dataMTrig_Audio_c__R.vi"() -> ("output_Audio_c__R"=w336:i32)  [unwired: 11 in]
      n200 = call "myRIO_BRig_RT_dataMTrig_Audio_Tcycle__R.vi"() -> ("output_Audio_Tcycle__R"=w337:i32)  [unwired: 11 in]
      n201 = Index Array(array=w356, index #1=w344, index #2=w350, index #3=w336, index #4=w337) -> (element #1=w349:u16, element #2=w348:u16, element #3=w339:u16, element #4=w338:u16)
      n202 = Add(x=w332, y=w349) -> (x+y=w353:u16)
      n203 = Add(x=w332, y=w339) -> (x+y=w342:u16)
      n204 = Less?(x=w353, y=w348) -> (x < y?=w330:bool)
      n205 = Less?(x=w342, y=w338) -> (x < y?=w331:bool)
      n206 = Decrement(x=w351) -> (x-1=w354:u16)
      n207 = Decrement(x=w340) -> (x-1=w343:u16)
      n208 = Select(t=w353, s=w330, f=u16 0) -> (s? t:f=w347:u16)
      n209 = Select(t=w351, s=w330, f=w354) -> (s? t:f=w346:u16)
      n210 = Select(t=w342, s=w331, f=u16 0) -> (s? t:f=w334:u16)
      n211 = Select(t=w340, s=w331, f=w343) -> (s? t:f=w333:u16)
      n212 = Replace Array Subset(array=w356, new element #1=w347, index #1=w344, new element #2=w346, index #2=w345, new element #3=w334, index #3=w336, new element #4=w333, index #4=w335) -> (w355:u16[])
    }
    frame 13 {
      # "Audio_R"
      # "Tcycle"
      # "count"
      # "Audio_L"
      # "Tcycle"
      # "count"
      # "Solenoid__L"
      # "Tcycle"
      # "count"
      n213 = call "myRIO_BRig_RT_dataMTrig_Solenoid_c__L.vi"() -> ("output_Solenoid_c__L"=w360:i32)  [unwired: 11 in]
      n214 = call "myRIO_BRig_RT_dataMTrig_Solenoid_Tcycle__L.vi"() -> ("output_Solenoid_Tcycle__L"=w363:i32)  [unwired: 11 in]
      n215 = call "myRIO_BRig_RT_dataMTrig_Audio_c__L.vi"() -> ("output_Audio_c__L"=w379:i32)  [unwired: 11 in]
      n216 = call "myRIO_BRig_RT_dataMTrig_Audio_Tcycle__L.vi"() -> ("output_Audio_Tcycle__L"=w385:i32)  [unwired: 11 in]
      n217 = call "myRIO_BRig_RT_dataMTrig_Audio_c__R.vi"() -> ("output_Audio_c__R"=w371:i32)  [unwired: 11 in]
      n218 = call "myRIO_BRig_RT_dataMTrig_Audio_Tcycle__R.vi"() -> ("output_Audio_Tcycle__R"=w372:i32)  [unwired: 11 in]
      n219 = Index Array(array=w392, index #1=w360, index #2=w363, index #3=w379, index #4=w385, index #5=w371, index #6=w372) -> (element #1=w362:u16, element #2=w361:u16, element #3=w384:u16, element #4=w383:u16, element #5=w374:u16, element #6=w373:u16)
      n220 = Add(x=w367, y=w362) -> (x+y=w394:u16)
      n221 = Add(x=w367, y=w384) -> (x+y=w388:u16)
      n222 = Add(x=w367, y=w374) -> (x+y=w377:u16)
      n223 = Less?(x=w394, y=w361) -> (x < y?=w364:bool)
      n224 = Less?(x=w388, y=w383) -> (x < y?=w365:bool)
      n225 = Less?(x=w377, y=w373) -> (x < y?=w366:bool)
      n226 = Decrement(x=w391) -> (x-1=w395:u16)
      n227 = Decrement(x=w386) -> (x-1=w389:u16)
      n228 = Decrement(x=w375) -> (x-1=w378:u16)
      n229 = Select(t=w394, s=w364, f=u16 0) -> (s? t:f=w359:u16)
      n230 = Select(t=w391, s=w364, f=w395) -> (s? t:f=w357:u16)
      n231 = Select(t=w388, s=w365, f=u16 0) -> (s? t:f=w382:u16)
      n232 = Select(t=w386, s=w365, f=w389) -> (s? t:f=w381:u16)
      n233 = Select(t=w377, s=w366, f=u16 0) -> (s? t:f=w369:u16)
      n234 = Select(t=w375, s=w366, f=w378) -> (s? t:f=w368:u16)
      n235 = Replace Array Subset(array=w392, new element #1=w359, index #1=w360, new element #2=w357, index #2=w358, new element #3=w382, index #3=w379, new element #4=w381, index #4=w380, new element #5=w369, index #5=w371, new element #6=w368, index #6=w370) -> (w390:u16[])
    }
    frame 14 {
      # "Audio_R"
      # "Tcycle"
      # "count"
      # "Audio_L"
      # "Tcycle"
      # "count"
      # "Solenoid__R"
      # "Tcycle"
      # "count"
      n236 = call "myRIO_BRig_RT_dataMTrig_Solenoid_c__R.vi"() -> ("output_Solenoid_c__R"=w426:i32)  [unwired: 11 in]
      n237 = call "myRIO_BRig_RT_dataMTrig_Solenoid_Tcycle__R.vi"() -> ("output_Solenoid_Tcycle__R"=w429:i32)  [unwired: 11 in]
      n238 = call "myRIO_BRig_RT_dataMTrig_Audio_c__L.vi"() -> ("output_Audio_c__L"=w411:i32)  [unwired: 11 in]
      n239 = call "myRIO_BRig_RT_dataMTrig_Audio_Tcycle__L.vi"() -> ("output_Audio_Tcycle__L"=w417:i32)  [unwired: 11 in]
      n240 = call "myRIO_BRig_RT_dataMTrig_Audio_c__R.vi"() -> ("output_Audio_c__R"=w403:i32)  [unwired: 11 in]
      n241 = call "myRIO_BRig_RT_dataMTrig_Audio_Tcycle__R.vi"() -> ("output_Audio_Tcycle__R"=w404:i32)  [unwired: 11 in]
      n242 = Index Array(array=w434, index #1=w426, index #2=w429, index #3=w411, index #4=w417, index #5=w403, index #6=w404) -> (element #1=w428:u16, element #2=w427:u16, element #3=w416:u16, element #4=w415:u16, element #5=w406:u16, element #6=w405:u16)
      n243 = Add(x=w399, y=w428) -> (x+y=w432:u16)
      n244 = Add(x=w399, y=w416) -> (x+y=w420:u16)
      n245 = Add(x=w399, y=w406) -> (x+y=w409:u16)
      n246 = Less?(x=w432, y=w427) -> (x < y?=w396:bool)
      n247 = Less?(x=w420, y=w415) -> (x < y?=w397:bool)
      n248 = Less?(x=w409, y=w405) -> (x < y?=w398:bool)
      n249 = Decrement(x=w430) -> (x-1=w433:u16)
      n250 = Decrement(x=w418) -> (x-1=w421:u16)
      n251 = Decrement(x=w407) -> (x-1=w410:u16)
      n252 = Select(t=w432, s=w396, f=u16 0) -> (s? t:f=w425:u16)
      n253 = Select(t=w430, s=w396, f=w433) -> (s? t:f=w423:u16)
      n254 = Select(t=w420, s=w397, f=u16 0) -> (s? t:f=w414:u16)
      n255 = Select(t=w418, s=w397, f=w421) -> (s? t:f=w413:u16)
      n256 = Select(t=w409, s=w398, f=u16 0) -> (s? t:f=w401:u16)
      n257 = Select(t=w407, s=w398, f=w410) -> (s? t:f=w400:u16)
      n258 = Replace Array Subset(array=w434, new element #1=w425, index #1=w426, new element #2=w423, index #2=w424, new element #3=w414, index #3=w411, new element #4=w413, index #4=w412, new element #5=w401, index #5=w403, new element #6=w400, index #6=w402) -> (w422:u16[])
    }
    frame 15 {
      # "Audio_R"
      # "Tcycle"
      # "count"
      # "Audio_L"
      # "Tcycle"
      # "count"
      # "Solenoid__R"
      # "Tcycle"
      # "count"
      # "Solenoid__L"
      # "Tcycle"
      # "count"
      n259 = call "myRIO_BRig_RT_dataMTrig_Solenoid_c__L.vi"() -> ("output_Solenoid_c__L"=w474:i32)  [unwired: 11 in]
      n260 = call "myRIO_BRig_RT_dataMTrig_Solenoid_Tcycle__L.vi"() -> ("output_Solenoid_Tcycle__L"=w485:i32)  [unwired: 11 in]
      n261 = call "myRIO_BRig_RT_dataMTrig_Solenoid_c__R.vi"() -> ("output_Solenoid_c__R"=w466:i32)  [unwired: 11 in]
      n262 = call "myRIO_BRig_RT_dataMTrig_Solenoid_Tcycle__R.vi"() -> ("output_Solenoid_Tcycle__R"=w469:i32)  [unwired: 11 in]
      n263 = call "myRIO_BRig_RT_dataMTrig_Audio_c__L.vi"() -> ("output_Audio_c__L"=w451:i32)  [unwired: 11 in]
      n264 = call "myRIO_BRig_RT_dataMTrig_Audio_Tcycle__L.vi"() -> ("output_Audio_Tcycle__L"=w457:i32)  [unwired: 11 in]
      n265 = call "myRIO_BRig_RT_dataMTrig_Audio_c__R.vi"() -> ("output_Audio_c__R"=w443:i32)  [unwired: 11 in]
      n266 = call "myRIO_BRig_RT_dataMTrig_Audio_Tcycle__R.vi"() -> ("output_Audio_Tcycle__R"=w444:i32)  [unwired: 11 in]
      n267 = Index Array(array=w479, index #1=w474, index #2=w485, index #3=w466, index #4=w469, index #5=w451, index #6=w457, index #7=w443, index #8=w444) -> (element #1=w484:u16, element #2=w483:u16, element #3=w468:u16, element #4=w467:u16, element #5=w456:u16, element #6=w455:u16, element #7=w446:u16, element #8=w445:u16)
      n268 = Add(x=w439, y=w484) -> (x+y=w481:u16)
      n269 = Add(x=w439, y=w468) -> (x+y=w472:u16)
      n270 = Add(x=w439, y=w456) -> (x+y=w460:u16)
      n271 = Add(x=w439, y=w446) -> (x+y=w449:u16)
      n272 = Less?(x=w481, y=w483) -> (x < y?=w435:bool)
      n273 = Less?(x=w472, y=w467) -> (x < y?=w436:bool)
      n274 = Less?(x=w460, y=w455) -> (x < y?=w437:bool)
      n275 = Less?(x=w449, y=w445) -> (x < y?=w438:bool)
      n276 = Decrement(x=w476) -> (x-1=w482:u16)
      n277 = Decrement(x=w470) -> (x-1=w473:u16)
      n278 = Decrement(x=w458) -> (x-1=w461:u16)
      n279 = Decrement(x=w447) -> (x-1=w450:u16)
      n280 = Select(t=w481, s=w435, f=u16 0) -> (s? t:f=w477:u16)
      n281 = Select(t=w476, s=w435, f=w482) -> (s? t:f=w478:u16)
      n282 = Select(t=w472, s=w436, f=u16 0) -> (s? t:f=w465:u16)
      n283 = Select(t=w470, s=w436, f=w473) -> (s? t:f=w463:u16)
      n284 = Select(t=w460, s=w437, f=u16 0) -> (s? t:f=w454:u16)
      n285 = Select(t=w458, s=w437, f=w461) -> (s? t:f=w453:u16)
      n286 = Select(t=w449, s=w438, f=u16 0) -> (s? t:f=w441:u16)
      n287 = Select(t=w447, s=w438, f=w450) -> (s? t:f=w440:u16)
      n288 = Replace Array Subset(array=w479, new element #1=w477, index #1=w474, new element #2=w478, index #2=w475, new element #3=w465, index #3=w466, new element #4=w463, index #4=w464, new element #5=w454, index #5=w451, new element #6=w453, index #6=w452, new element #7=w441, index #7=w443, new element #8=w440, index #8=w442) -> (w462:u16[])
    }
    frame 16 {
      # "Laser"
      # "Tcycle"
      # "count"
      n289 = call "myRIO_BRig_RT_dataMTrig_Laser_c.vi"() -> ("output_Laser_c"=w490:i32)  [unwired: 11 in]
      n290 = call "myRIO_BRig_RT_dataMTrig_Laser_Tcycle.vi"() -> ("output_Laser_Tcycle"=w493:i32)  [unwired: 11 in]
      n291 = Index Array(array=w500, index #1=w490, index #2=w493) -> (element #1=w492:u16, element #2=w491:u16)
      n292 = Add(x=w494, y=w492) -> (x+y=w497:u16)
      n293 = Less?(x=w497, y=w491) -> (x < y?=w486:bool)
      n294 = Decrement(x=w495) -> (x-1=w498:u16)
      n295 = Select(t=w497, s=w486, f=u16 0) -> (s? t:f=w488:u16)
      n296 = Select(t=w495, s=w486, f=w498) -> (s? t:f=w487:u16)
      n297 = Replace Array Subset(array=w500, new element #1=w488, index #1=w490, new element #2=w487, index #2=w489) -> (w499:u16[])
    }
    frame 17 {
      # "Laser"
      # "Tcycle"
      # "count"
      # "Solenoid__L"
      # "Tcycle"
      # "count"
      n298 = call "myRIO_BRig_RT_dataMTrig_Solenoid_c__L.vi"() -> ("output_Solenoid_c__L"=w516:i32)  [unwired: 11 in]
      n299 = call "myRIO_BRig_RT_dataMTrig_Solenoid_Tcycle__L.vi"() -> ("output_Solenoid_Tcycle__L"=w527:i32)  [unwired: 11 in]
      n300 = call "myRIO_BRig_RT_dataMTrig_Laser_c.vi"() -> ("output_Laser_c"=w504:i32)  [unwired: 11 in]
      n301 = call "myRIO_BRig_RT_dataMTrig_Laser_Tcycle.vi"() -> ("output_Laser_Tcycle"=w507:i32)  [unwired: 11 in]
      n302 = Index Array(array=w521, index #1=w516, index #2=w527, index #3=w504, index #4=w507) -> (element #1=w526:u16, element #2=w525:u16, element #3=w506:u16, element #4=w505:u16)
      n303 = Add(x=w510, y=w526) -> (x+y=w523:u16)
      n304 = Add(x=w510, y=w506) -> (x+y=w513:u16)
      n305 = Less?(x=w523, y=w525) -> (x < y?=w508:bool)
      n306 = Less?(x=w513, y=w505) -> (x < y?=w509:bool)
      n307 = Decrement(x=w518) -> (x-1=w524:u16)
      n308 = Decrement(x=w511) -> (x-1=w514:u16)
      n309 = Select(t=w523, s=w508, f=u16 0) -> (s? t:f=w519:u16)
      n310 = Select(t=w518, s=w508, f=w524) -> (s? t:f=w520:u16)
      n311 = Select(t=w513, s=w509, f=u16 0) -> (s? t:f=w503:u16)
      n312 = Select(t=w511, s=w509, f=w514) -> (s? t:f=w501:u16)
      n313 = Replace Array Subset(array=w521, new element #1=w519, index #1=w516, new element #2=w520, index #2=w517, new element #3=w503, index #3=w504, new element #4=w501, index #4=w502) -> (w515:u16[])
    }
    frame 18 {
      # "Laser"
      # "Tcycle"
      # "count"
      # "Solenoid__R"
      # "Tcycle"
      # "count"
      n314 = call "myRIO_BRig_RT_dataMTrig_Solenoid_c__R.vi"() -> ("output_Solenoid_c__R"=w546:i32)  [unwired: 11 in]
      n315 = call "myRIO_BRig_RT_dataMTrig_Solenoid_Tcycle__R.vi"() -> ("output_Solenoid_Tcycle__R"=w549:i32)  [unwired: 11 in]
      n316 = call "myRIO_BRig_RT_dataMTrig_Laser_c.vi"() -> ("output_Laser_c"=w531:i32)  [unwired: 11 in]
      n317 = call "myRIO_BRig_RT_dataMTrig_Laser_Tcycle.vi"() -> ("output_Laser_Tcycle"=w534:i32)  [unwired: 11 in]
      n318 = Index Array(array=w554, index #1=w546, index #2=w549, index #3=w531, index #4=w534) -> (element #1=w548:u16, element #2=w547:u16, element #3=w533:u16, element #4=w532:u16)
      n319 = Add(x=w537, y=w548) -> (x+y=w552:u16)
      n320 = Add(x=w537, y=w533) -> (x+y=w540:u16)
      n321 = Less?(x=w552, y=w547) -> (x < y?=w535:bool)
      n322 = Less?(x=w540, y=w532) -> (x < y?=w536:bool)
      n323 = Decrement(x=w550) -> (x-1=w553:u16)
      n324 = Decrement(x=w538) -> (x-1=w541:u16)
      n325 = Select(t=w552, s=w535, f=u16 0) -> (s? t:f=w545:u16)
      n326 = Select(t=w550, s=w535, f=w553) -> (s? t:f=w543:u16)
      n327 = Select(t=w540, s=w536, f=u16 0) -> (s? t:f=w530:u16)
      n328 = Select(t=w538, s=w536, f=w541) -> (s? t:f=w528:u16)
      n329 = Replace Array Subset(array=w554, new element #1=w545, index #1=w546, new element #2=w543, index #2=w544, new element #3=w530, index #3=w531, new element #4=w528, index #4=w529) -> (w542:u16[])
    }
    frame 19 {
      # "Laser"
      # "Tcycle"
      # "count"
      # "Solenoid__R"
      # "Tcycle"
      # "count"
      # "Solenoid__L"
      # "Tcycle"
      # "count"
      n330 = call "myRIO_BRig_RT_dataMTrig_Solenoid_c__L.vi"() -> ("output_Solenoid_c__L"=w582:i32)  [unwired: 11 in]
      n331 = call "myRIO_BRig_RT_dataMTrig_Solenoid_Tcycle__L.vi"() -> ("output_Solenoid_Tcycle__L"=w593:i32)  [unwired: 11 in]
      n332 = call "myRIO_BRig_RT_dataMTrig_Solenoid_c__R.vi"() -> ("output_Solenoid_c__R"=w574:i32)  [unwired: 11 in]
      n333 = call "myRIO_BRig_RT_dataMTrig_Solenoid_Tcycle__R.vi"() -> ("output_Solenoid_Tcycle__R"=w577:i32)  [unwired: 11 in]
      n334 = call "myRIO_BRig_RT_dataMTrig_Laser_c.vi"() -> ("output_Laser_c"=w558:i32)  [unwired: 11 in]
      n335 = call "myRIO_BRig_RT_dataMTrig_Laser_Tcycle.vi"() -> ("output_Laser_Tcycle"=w561:i32)  [unwired: 11 in]
      n336 = Index Array(array=w587, index #1=w582, index #2=w593, index #3=w574, index #4=w577, index #5=w558, index #6=w561) -> (element #1=w592:u16, element #2=w591:u16, element #3=w576:u16, element #4=w575:u16, element #5=w560:u16, element #6=w559:u16)
      n337 = Add(x=w565, y=w592) -> (x+y=w589:u16)
      n338 = Add(x=w565, y=w576) -> (x+y=w580:u16)
      n339 = Add(x=w565, y=w560) -> (x+y=w568:u16)
      n340 = Less?(x=w589, y=w591) -> (x < y?=w562:bool)
      n341 = Less?(x=w580, y=w575) -> (x < y?=w563:bool)
      n342 = Less?(x=w568, y=w559) -> (x < y?=w564:bool)
      n343 = Decrement(x=w584) -> (x-1=w590:u16)
      n344 = Decrement(x=w578) -> (x-1=w581:u16)
      n345 = Decrement(x=w566) -> (x-1=w569:u16)
      n346 = Select(t=w589, s=w562, f=u16 0) -> (s? t:f=w585:u16)
      n347 = Select(t=w584, s=w562, f=w590) -> (s? t:f=w586:u16)
      n348 = Select(t=w580, s=w563, f=u16 0) -> (s? t:f=w573:u16)
      n349 = Select(t=w578, s=w563, f=w581) -> (s? t:f=w571:u16)
      n350 = Select(t=w568, s=w564, f=u16 0) -> (s? t:f=w557:u16)
      n351 = Select(t=w566, s=w564, f=w569) -> (s? t:f=w555:u16)
      n352 = Replace Array Subset(array=w587, new element #1=w585, index #1=w582, new element #2=w586, index #2=w583, new element #3=w573, index #3=w574, new element #4=w571, index #4=w572, new element #5=w557, index #5=w558, new element #6=w555, index #6=w556) -> (w570:u16[])
    }
    frame 20 {
      # "Laser"
      # "Tcycle"
      # "count"
      # "Audio_L"
      # "Tcycle"
      # "count"
      n353 = call "myRIO_BRig_RT_dataMTrig_Audio_c__L.vi"() -> ("output_Audio_c__L"=w608:i32)  [unwired: 11 in]
      n354 = call "myRIO_BRig_RT_dataMTrig_Audio_Tcycle__L.vi"() -> ("output_Audio_Tcycle__L"=w614:i32)  [unwired: 11 in]
      n355 = call "myRIO_BRig_RT_dataMTrig_Laser_c.vi"() -> ("output_Laser_c"=w597:i32)  [unwired: 11 in]
      n356 = call "myRIO_BRig_RT_dataMTrig_Laser_Tcycle.vi"() -> ("output_Laser_Tcycle"=w600:i32)  [unwired: 11 in]
      n357 = Index Array(array=w620, index #1=w608, index #2=w614, index #3=w597, index #4=w600) -> (element #1=w613:u16, element #2=w612:u16, element #3=w599:u16, element #4=w598:u16)
      n358 = Add(x=w603, y=w613) -> (x+y=w617:u16)
      n359 = Add(x=w603, y=w599) -> (x+y=w606:u16)
      n360 = Less?(x=w617, y=w612) -> (x < y?=w601:bool)
      n361 = Less?(x=w606, y=w598) -> (x < y?=w602:bool)
      n362 = Decrement(x=w615) -> (x-1=w618:u16)
      n363 = Decrement(x=w604) -> (x-1=w607:u16)
      n364 = Select(t=w617, s=w601, f=u16 0) -> (s? t:f=w611:u16)
      n365 = Select(t=w615, s=w601, f=w618) -> (s? t:f=w610:u16)
      n366 = Select(t=w606, s=w602, f=u16 0) -> (s? t:f=w596:u16)
      n367 = Select(t=w604, s=w602, f=w607) -> (s? t:f=w594:u16)
      n368 = Replace Array Subset(array=w620, new element #1=w611, index #1=w608, new element #2=w610, index #2=w609, new element #3=w596, index #3=w597, new element #4=w594, index #4=w595) -> (w619:u16[])
    }
    frame 21 {
      # "Laser"
      # "Tcycle"
      # "count"
      # "Audio_L"
      # "Tcycle"
      # "count"
      # "Solenoid__L"
      # "Tcycle"
      # "count"
      n369 = call "myRIO_BRig_RT_dataMTrig_Solenoid_c__L.vi"() -> ("output_Solenoid_c__L"=w648:i32)  [unwired: 11 in]
      n370 = call "myRIO_BRig_RT_dataMTrig_Solenoid_Tcycle__L.vi"() -> ("output_Solenoid_Tcycle__L"=w659:i32)  [unwired: 11 in]
      n371 = call "myRIO_BRig_RT_dataMTrig_Audio_c__L.vi"() -> ("output_Audio_c__L"=w628:i32)  [unwired: 11 in]
      n372 = call "myRIO_BRig_RT_dataMTrig_Audio_Tcycle__L.vi"() -> ("output_Audio_Tcycle__L"=w634:i32)  [unwired: 11 in]
      n373 = call "myRIO_BRig_RT_dataMTrig_Laser_c.vi"() -> ("output_Laser_c"=w624:i32)  [unwired: 11 in]
      n374 = call "myRIO_BRig_RT_dataMTrig_Laser_Tcycle.vi"() -> ("output_Laser_Tcycle"=w633:i32)  [unwired: 11 in]
      n375 = Index Array(array=w653, index #1=w648, index #2=w659, index #3=w628, index #4=w634, index #5=w624, index #6=w633) -> (element #1=w658:u16, element #2=w657:u16, element #3=w632:u16, element #4=w631:u16, element #5=w630:u16, element #6=w629:u16)
      n376 = Add(x=w638, y=w658) -> (x+y=w655:u16)
      n377 = Add(x=w638, y=w632) -> (x+y=w645:u16)
      n378 = Add(x=w638, y=w630) -> (x+y=w641:u16)
      n379 = Less?(x=w655, y=w657) -> (x < y?=w635:bool)
      n380 = Less?(x=w645, y=w631) -> (x < y?=w636:bool)
      n381 = Less?(x=w641, y=w629) -> (x < y?=w637:bool)
      n382 = Decrement(x=w650) -> (x-1=w656:u16)
      n383 = Decrement(x=w643) -> (x-1=w646:u16)
      n384 = Decrement(x=w639) -> (x-1=w642:u16)
      n385 = Select(t=w655, s=w635, f=u16 0) -> (s? t:f=w651:u16)
      n386 = Select(t=w650, s=w635, f=w656) -> (s? t:f=w652:u16)
      n387 = Select(t=w645, s=w636, f=u16 0) -> (s? t:f=w627:u16)
      n388 = Select(t=w643, s=w636, f=w646) -> (s? t:f=w625:u16)
      n389 = Select(t=w641, s=w637, f=u16 0) -> (s? t:f=w623:u16)
      n390 = Select(t=w639, s=w637, f=w642) -> (s? t:f=w621:u16)
      n391 = Replace Array Subset(array=w653, new element #1=w651, index #1=w648, new element #2=w652, index #2=w649, new element #3=w627, index #3=w628, new element #4=w625, index #4=w626, new element #5=w623, index #5=w624, new element #6=w621, index #6=w622) -> (w647:u16[])
    }
    frame 22 {
      # "Laser"
      # "Tcycle"
      # "count"
      # "Audio_L"
      # "Tcycle"
      # "count"
      # "Solenoid__R"
      # "Tcycle"
      # "count"
      n392 = call "myRIO_BRig_RT_dataMTrig_Solenoid_c__R.vi"() -> ("output_Solenoid_c__R"=w690:i32)  [unwired: 11 in]
      n393 = call "myRIO_BRig_RT_dataMTrig_Solenoid_Tcycle__R.vi"() -> ("output_Solenoid_Tcycle__R"=w693:i32)  [unwired: 11 in]
      n394 = call "myRIO_BRig_RT_dataMTrig_Audio_c__L.vi"() -> ("output_Audio_c__L"=w675:i32)  [unwired: 11 in]
      n395 = call "myRIO_BRig_RT_dataMTrig_Audio_Tcycle__L.vi"() -> ("output_Audio_Tcycle__L"=w681:i32)  [unwired: 11 in]
      n396 = call "myRIO_BRig_RT_dataMTrig_Laser_c.vi"() -> ("output_Laser_c"=w663:i32)  [unwired: 11 in]
      n397 = call "myRIO_BRig_RT_dataMTrig_Laser_Tcycle.vi"() -> ("output_Laser_Tcycle"=w666:i32)  [unwired: 11 in]
      n398 = Index Array(array=w698, index #1=w690, index #2=w693, index #3=w675, index #4=w681, index #5=w663, index #6=w666) -> (element #1=w692:u16, element #2=w691:u16, element #3=w680:u16, element #4=w679:u16, element #5=w665:u16, element #6=w664:u16)
      n399 = Add(x=w670, y=w692) -> (x+y=w696:u16)
      n400 = Add(x=w670, y=w680) -> (x+y=w684:u16)
      n401 = Add(x=w670, y=w665) -> (x+y=w673:u16)
      n402 = Less?(x=w696, y=w691) -> (x < y?=w667:bool)
      n403 = Less?(x=w684, y=w679) -> (x < y?=w668:bool)
      n404 = Less?(x=w673, y=w664) -> (x < y?=w669:bool)
      n405 = Decrement(x=w694) -> (x-1=w697:u16)
      n406 = Decrement(x=w682) -> (x-1=w685:u16)
      n407 = Decrement(x=w671) -> (x-1=w674:u16)
      n408 = Select(t=w696, s=w667, f=u16 0) -> (s? t:f=w689:u16)
      n409 = Select(t=w694, s=w667, f=w697) -> (s? t:f=w687:u16)
      n410 = Select(t=w684, s=w668, f=u16 0) -> (s? t:f=w678:u16)
      n411 = Select(t=w682, s=w668, f=w685) -> (s? t:f=w677:u16)
      n412 = Select(t=w673, s=w669, f=u16 0) -> (s? t:f=w662:u16)
      n413 = Select(t=w671, s=w669, f=w674) -> (s? t:f=w660:u16)
      n414 = Replace Array Subset(array=w698, new element #1=w689, index #1=w690, new element #2=w687, index #2=w688, new element #3=w678, index #3=w675, new element #4=w677, index #4=w676, new element #5=w662, index #5=w663, new element #6=w660, index #6=w661) -> (w686:u16[])
    }
    frame 23 {
      # "Laser"
      # "Tcycle"
      # "count"
      # "Audio_L"
      # "Tcycle"
      # "count"
      # "Solenoid__R"
      # "Tcycle"
      # "count"
      # "Solenoid__L"
      # "Tcycle"
      # "count"
      n415 = call "myRIO_BRig_RT_dataMTrig_Solenoid_c__L.vi"() -> ("output_Solenoid_c__L"=w738:i32)  [unwired: 11 in]
      n416 = call "myRIO_BRig_RT_dataMTrig_Solenoid_Tcycle__L.vi"() -> ("output_Solenoid_Tcycle__L"=w749:i32)  [unwired: 11 in]
      n417 = call "myRIO_BRig_RT_dataMTrig_Solenoid_c__R.vi"() -> ("output_Solenoid_c__R"=w730:i32)  [unwired: 11 in]
      n418 = call "myRIO_BRig_RT_dataMTrig_Solenoid_Tcycle__R.vi"() -> ("output_Solenoid_Tcycle__R"=w733:i32)  [unwired: 11 in]
      n419 = call "myRIO_BRig_RT_dataMTrig_Audio_c__L.vi"() -> ("output_Audio_c__L"=w715:i32)  [unwired: 11 in]
      n420 = call "myRIO_BRig_RT_dataMTrig_Audio_Tcycle__L.vi"() -> ("output_Audio_Tcycle__L"=w721:i32)  [unwired: 11 in]
      n421 = call "myRIO_BRig_RT_dataMTrig_Laser_c.vi"() -> ("output_Laser_c"=w702:i32)  [unwired: 11 in]
      n422 = call "myRIO_BRig_RT_dataMTrig_Laser_Tcycle.vi"() -> ("output_Laser_Tcycle"=w705:i32)  [unwired: 11 in]
      n423 = Index Array(array=w743, index #1=w738, index #2=w749, index #3=w730, index #4=w733, index #5=w715, index #6=w721, index #7=w702, index #8=w705) -> (element #1=w748:u16, element #2=w747:u16, element #3=w732:u16, element #4=w731:u16, element #5=w720:u16, element #6=w719:u16, element #7=w704:u16, element #8=w703:u16)
      n424 = Add(x=w710, y=w748) -> (x+y=w745:u16)
      n425 = Add(x=w710, y=w732) -> (x+y=w736:u16)
      n426 = Add(x=w710, y=w720) -> (x+y=w724:u16)
      n427 = Add(x=w710, y=w704) -> (x+y=w713:u16)
      n428 = Less?(x=w745, y=w747) -> (x < y?=w706:bool)
      n429 = Less?(x=w736, y=w731) -> (x < y?=w707:bool)
      n430 = Less?(x=w724, y=w719) -> (x < y?=w708:bool)
      n431 = Less?(x=w713, y=w703) -> (x < y?=w709:bool)
      n432 = Decrement(x=w740) -> (x-1=w746:u16)
      n433 = Decrement(x=w734) -> (x-1=w737:u16)
      n434 = Decrement(x=w722) -> (x-1=w725:u16)
      n435 = Decrement(x=w711) -> (x-1=w714:u16)
      n436 = Select(t=w745, s=w706, f=u16 0) -> (s? t:f=w741:u16)
      n437 = Select(t=w740, s=w706, f=w746) -> (s? t:f=w742:u16)
      n438 = Select(t=w736, s=w707, f=u16 0) -> (s? t:f=w729:u16)
      n439 = Select(t=w734, s=w707, f=w737) -> (s? t:f=w727:u16)
      n440 = Select(t=w724, s=w708, f=u16 0) -> (s? t:f=w718:u16)
      n441 = Select(t=w722, s=w708, f=w725) -> (s? t:f=w717:u16)
      n442 = Select(t=w713, s=w709, f=u16 0) -> (s? t:f=w701:u16)
      n443 = Select(t=w711, s=w709, f=w714) -> (s? t:f=w699:u16)
      n444 = Replace Array Subset(array=w743, new element #1=w741, index #1=w738, new element #2=w742, index #2=w739, new element #3=w729, index #3=w730, new element #4=w727, index #4=w728, new element #5=w718, index #5=w715, new element #6=w717, index #6=w716, new element #7=w701, index #7=w702, new element #8=w699, index #8=w700) -> (w726:u16[])
    }
    frame 24 {
      # "Laser"
      # "Tcycle"
      # "count"
      # "Audio_R"
      # "Tcycle"
      # "count"
      n445 = call "myRIO_BRig_RT_dataMTrig_Audio_c__R.vi"() -> ("output_Audio_c__R"=w767:i32)  [unwired: 11 in]
      n446 = call "myRIO_BRig_RT_dataMTrig_Audio_Tcycle__R.vi"() -> ("output_Audio_Tcycle__R"=w768:i32)  [unwired: 11 in]
      n447 = call "myRIO_BRig_RT_dataMTrig_Laser_c.vi"() -> ("output_Laser_c"=w755:i32)  [unwired: 11 in]
      n448 = call "myRIO_BRig_RT_dataMTrig_Laser_Tcycle.vi"() -> ("output_Laser_Tcycle"=w758:i32)  [unwired: 11 in]
      n449 = Index Array(array=w776, index #1=w767, index #2=w768, index #3=w755, index #4=w758) -> (element #1=w770:u16, element #2=w769:u16, element #3=w757:u16, element #4=w756:u16)
      n450 = Add(x=w759, y=w770) -> (x+y=w773:u16)
      n451 = Add(x=w759, y=w757) -> (x+y=w762:u16)
      n452 = Less?(x=w773, y=w769) -> (x < y?=w750:bool)
      n453 = Less?(x=w762, y=w756) -> (x < y?=w751:bool)
      n454 = Decrement(x=w771) -> (x-1=w774:u16)
      n455 = Decrement(x=w760) -> (x-1=w763:u16)
      n456 = Select(t=w773, s=w750, f=u16 0) -> (s? t:f=w765:u16)
      n457 = Select(t=w771, s=w750, f=w774) -> (s? t:f=w764:u16)
      n458 = Select(t=w762, s=w751, f=u16 0) -> (s? t:f=w753:u16)
      n459 = Select(t=w760, s=w751, f=w763) -> (s? t:f=w752:u16)
      n460 = Replace Array Subset(array=w776, new element #1=w765, index #1=w767, new element #2=w764, index #2=w766, new element #3=w753, index #3=w755, new element #4=w752, index #4=w754) -> (w775:u16[])
    }
    frame 25 {
      # "Laser"
      # "Tcycle"
      # "count"
      # "Audio_R"
      # "Tcycle"
      # "count"
      # "Solenoid__L"
      # "Tcycle"
      # "count"
      n461 = call "myRIO_BRig_RT_dataMTrig_Solenoid_c__L.vi"() -> ("output_Solenoid_c__L"=w780:i32)  [unwired: 11 in]
      n462 = call "myRIO_BRig_RT_dataMTrig_Solenoid_Tcycle__L.vi"() -> ("output_Solenoid_Tcycle__L"=w783:i32)  [unwired: 11 in]
      n463 = call "myRIO_BRig_RT_dataMTrig_Audio_c__R.vi"() -> ("output_Audio_c__R"=w802:i32)  [unwired: 11 in]
      n464 = call "myRIO_BRig_RT_dataMTrig_Audio_Tcycle__R.vi"() -> ("output_Audio_Tcycle__R"=w803:i32)  [unwired: 11 in]
      n465 = call "myRIO_BRig_RT_dataMTrig_Laser_c.vi"() -> ("output_Laser_c"=w790:i32)  [unwired: 11 in]
      n466 = call "myRIO_BRig_RT_dataMTrig_Laser_Tcycle.vi"() -> ("output_Laser_Tcycle"=w793:i32)  [unwired: 11 in]
      n467 = Index Array(array=w812, index #1=w780, index #2=w783, index #3=w802, index #4=w803, index #5=w790, index #6=w793) -> (element #1=w782:u16, element #2=w781:u16, element #3=w805:u16, element #4=w804:u16, element #5=w792:u16, element #6=w791:u16)
      n468 = Add(x=w794, y=w782) -> (x+y=w814:u16)
      n469 = Add(x=w794, y=w805) -> (x+y=w808:u16)
      n470 = Add(x=w794, y=w792) -> (x+y=w797:u16)
      n471 = Less?(x=w814, y=w781) -> (x < y?=w784:bool)
      n472 = Less?(x=w808, y=w804) -> (x < y?=w785:bool)
      n473 = Less?(x=w797, y=w791) -> (x < y?=w786:bool)
      n474 = Decrement(x=w811) -> (x-1=w815:u16)
      n475 = Decrement(x=w806) -> (x-1=w809:u16)
      n476 = Decrement(x=w795) -> (x-1=w798:u16)
      n477 = Select(t=w814, s=w784, f=u16 0) -> (s? t:f=w779:u16)
      n478 = Select(t=w811, s=w784, f=w815) -> (s? t:f=w777:u16)
      n479 = Select(t=w808, s=w785, f=u16 0) -> (s? t:f=w800:u16)
      n480 = Select(t=w806, s=w785, f=w809) -> (s? t:f=w799:u16)
      n481 = Select(t=w797, s=w786, f=u16 0) -> (s? t:f=w788:u16)
      n482 = Select(t=w795, s=w786, f=w798) -> (s? t:f=w787:u16)
      n483 = Replace Array Subset(array=w812, new element #1=w779, index #1=w780, new element #2=w777, index #2=w778, new element #3=w800, index #3=w802, new element #4=w799, index #4=w801, new element #5=w788, index #5=w790, new element #6=w787, index #6=w789) -> (w810:u16[])
    }
    frame 26 {
      # "Laser"
      # "Tcycle"
      # "count"
      # "Audio_R"
      # "Tcycle"
      # "count"
      # "Solenoid__R"
      # "Tcycle"
      # "count"
      n484 = call "myRIO_BRig_RT_dataMTrig_Solenoid_c__R.vi"() -> ("output_Solenoid_c__R"=w817:i32)  [unwired: 11 in]
      n485 = call "myRIO_BRig_RT_dataMTrig_Solenoid_Tcycle__R.vi"() -> ("output_Solenoid_Tcycle__R"=w816:i32)  [unwired: 11 in]
      n486 = call "myRIO_BRig_RT_dataMTrig_Audio_c__R.vi"() -> ("output_Audio_c__R"=w841:i32)  [unwired: 11 in]
      n487 = call "myRIO_BRig_RT_dataMTrig_Audio_Tcycle__R.vi"() -> ("output_Audio_Tcycle__R"=w842:i32)  [unwired: 11 in]
      n488 = call "myRIO_BRig_RT_dataMTrig_Laser_c.vi"() -> ("output_Laser_c"=w829:i32)  [unwired: 11 in]
      n489 = call "myRIO_BRig_RT_dataMTrig_Laser_Tcycle.vi"() -> ("output_Laser_Tcycle"=w832:i32)  [unwired: 11 in]
      n490 = Index Array(array=w854, index #1=w817, index #2=w816, index #3=w841, index #4=w842, index #5=w829, index #6=w832) -> (element #1=w819:u16, element #2=w818:u16, element #3=w844:u16, element #4=w843:u16, element #5=w831:u16, element #6=w830:u16)
      n491 = Add(x=w833, y=w819) -> (x+y=w852:u16)
      n492 = Add(x=w833, y=w844) -> (x+y=w847:u16)
      n493 = Add(x=w833, y=w831) -> (x+y=w836:u16)
      n494 = Less?(x=w852, y=w818) -> (x < y?=w823:bool)
      n495 = Less?(x=w847, y=w843) -> (x < y?=w824:bool)
      n496 = Less?(x=w836, y=w830) -> (x < y?=w825:bool)
      n497 = Decrement(x=w850) -> (x-1=w853:u16)
      n498 = Decrement(x=w845) -> (x-1=w848:u16)
      n499 = Decrement(x=w834) -> (x-1=w837:u16)
      n500 = Select(t=w852, s=w823, f=u16 0) -> (s? t:f=w822:u16)
      n501 = Select(t=w850, s=w823, f=w853) -> (s? t:f=w820:u16)
      n502 = Select(t=w847, s=w824, f=u16 0) -> (s? t:f=w839:u16)
      n503 = Select(t=w845, s=w824, f=w848) -> (s? t:f=w838:u16)
      n504 = Select(t=w836, s=w825, f=u16 0) -> (s? t:f=w827:u16)
      n505 = Select(t=w834, s=w825, f=w837) -> (s? t:f=w826:u16)
      n506 = Replace Array Subset(array=w854, new element #1=w822, index #1=w817, new element #2=w820, index #2=w821, new element #3=w839, index #3=w841, new element #4=w838, index #4=w840, new element #5=w827, index #5=w829, new element #6=w826, index #6=w828) -> (w849:u16[])
    }
    frame 27 {
      # "Laser"
      # "Tcycle"
      # "count"
      # "Audio_R"
      # "Tcycle"
      # "count"
      # "Solenoid__R"
      # "Tcycle"
      # "count"
      # "Solenoid__L"
      # "Tcycle"
      # "count"
      n507 = call "myRIO_BRig_RT_dataMTrig_Solenoid_c__L.vi"() -> ("output_Solenoid_c__L"=w894:i32)  [unwired: 11 in]
      n508 = call "myRIO_BRig_RT_dataMTrig_Solenoid_Tcycle__L.vi"() -> ("output_Solenoid_Tcycle__L"=w905:i32)  [unwired: 11 in]
      n509 = call "myRIO_BRig_RT_dataMTrig_Solenoid_c__R.vi"() -> ("output_Solenoid_c__R"=w886:i32)  [unwired: 11 in]
      n510 = call "myRIO_BRig_RT_dataMTrig_Solenoid_Tcycle__R.vi"() -> ("output_Solenoid_Tcycle__R"=w889:i32)  [unwired: 11 in]
      n511 = call "myRIO_BRig_RT_dataMTrig_Audio_c__R.vi"() -> ("output_Audio_c__R"=w862:i32)  [unwired: 11 in]
      n512 = call "myRIO_BRig_RT_dataMTrig_Audio_Tcycle__R.vi"() -> ("output_Audio_Tcycle__R"=w868:i32)  [unwired: 11 in]
      n513 = call "myRIO_BRig_RT_dataMTrig_Laser_c.vi"() -> ("output_Laser_c"=w858:i32)  [unwired: 11 in]
      n514 = call "myRIO_BRig_RT_dataMTrig_Laser_Tcycle.vi"() -> ("output_Laser_Tcycle"=w867:i32)  [unwired: 11 in]
      n515 = Index Array(array=w899, index #1=w894, index #2=w905, index #3=w886, index #4=w889, index #5=w862, index #6=w868, index #7=w858, index #8=w867) -> (element #1=w904:u16, element #2=w903:u16, element #3=w888:u16, element #4=w887:u16, element #5=w866:u16, element #6=w865:u16, element #7=w864:u16, element #8=w863:u16)
      n516 = Add(x=w873, y=w904) -> (x+y=w901:u16)
      n517 = Add(x=w873, y=w888) -> (x+y=w892:u16)
      n518 = Add(x=w873, y=w866) -> (x+y=w880:u16)
      n519 = Add(x=w873, y=w864) -> (x+y=w876:u16)
      n520 = Less?(x=w901, y=w903) -> (x < y?=w869:bool)
      n521 = Less?(x=w892, y=w887) -> (x < y?=w870:bool)
      n522 = Less?(x=w880, y=w865) -> (x < y?=w871:bool)
      n523 = Less?(x=w876, y=w863) -> (x < y?=w872:bool)
      n524 = Decrement(x=w896) -> (x-1=w902:u16)
      n525 = Decrement(x=w890) -> (x-1=w893:u16)
      n526 = Decrement(x=w878) -> (x-1=w881:u16)
      n527 = Decrement(x=w874) -> (x-1=w877:u16)
      n528 = Select(t=w901, s=w869, f=u16 0) -> (s? t:f=w897:u16)
      n529 = Select(t=w896, s=w869, f=w902) -> (s? t:f=w898:u16)
      n530 = Select(t=w892, s=w870, f=u16 0) -> (s? t:f=w885:u16)
      n531 = Select(t=w890, s=w870, f=w893) -> (s? t:f=w883:u16)
      n532 = Select(t=w880, s=w871, f=u16 0) -> (s? t:f=w861:u16)
      n533 = Select(t=w878, s=w871, f=w881) -> (s? t:f=w859:u16)
      n534 = Select(t=w876, s=w872, f=u16 0) -> (s? t:f=w857:u16)
      n535 = Select(t=w874, s=w872, f=w877) -> (s? t:f=w855:u16)
      n536 = Replace Array Subset(array=w899, new element #1=w897, index #1=w894, new element #2=w898, index #2=w895, new element #3=w885, index #3=w886, new element #4=w883, index #4=w884, new element #5=w861, index #5=w862, new element #6=w859, index #6=w860, new element #7=w857, index #7=w858, new element #8=w855, index #8=w856) -> (w882:u16[])
    }
    frame 28 {
      # "Laser"
      # "Tcycle"
      # "count"
      # "Audio_R"
      # "Tcycle"
      # "count"
      # "Audio_L"
      # "Tcycle"
      # "count"
      n537 = call "myRIO_BRig_RT_dataMTrig_Audio_c__L.vi"() -> ("output_Audio_c__L"=w932:i32)  [unwired: 11 in]
      n538 = call "myRIO_BRig_RT_dataMTrig_Audio_Tcycle__L.vi"() -> ("output_Audio_Tcycle__L"=w938:i32)  [unwired: 11 in]
      n539 = call "myRIO_BRig_RT_dataMTrig_Audio_c__R.vi"() -> ("output_Audio_c__R"=w924:i32)  [unwired: 11 in]
      n540 = call "myRIO_BRig_RT_dataMTrig_Audio_Tcycle__R.vi"() -> ("output_Audio_Tcycle__R"=w925:i32)  [unwired: 11 in]
      n541 = call "myRIO_BRig_RT_dataMTrig_Laser_c.vi"() -> ("output_Laser_c"=w912:i32)  [unwired: 11 in]
      n542 = call "myRIO_BRig_RT_dataMTrig_Laser_Tcycle.vi"() -> ("output_Laser_Tcycle"=w915:i32)  [unwired: 11 in]
      n543 = Index Array(array=w944, index #1=w932, index #2=w938, index #3=w924, index #4=w925, index #5=w912, index #6=w915) -> (element #1=w937:u16, element #2=w936:u16, element #3=w927:u16, element #4=w926:u16, element #5=w914:u16, element #6=w913:u16)
      n544 = Add(x=w916, y=w937) -> (x+y=w941:u16)
      n545 = Add(x=w916, y=w927) -> (x+y=w930:u16)
      n546 = Add(x=w916, y=w914) -> (x+y=w919:u16)
      n547 = Less?(x=w941, y=w936) -> (x < y?=w906:bool)
      n548 = Less?(x=w930, y=w926) -> (x < y?=w907:bool)
      n549 = Less?(x=w919, y=w913) -> (x < y?=w908:bool)
      n550 = Decrement(x=w939) -> (x-1=w942:u16)
      n551 = Decrement(x=w928) -> (x-1=w931:u16)
      n552 = Decrement(x=w917) -> (x-1=w920:u16)
      n553 = Select(t=w941, s=w906, f=u16 0) -> (s? t:f=w935:u16)
      n554 = Select(t=w939, s=w906, f=w942) -> (s? t:f=w934:u16)
      n555 = Select(t=w930, s=w907, f=u16 0) -> (s? t:f=w922:u16)
      n556 = Select(t=w928, s=w907, f=w931) -> (s? t:f=w921:u16)
      n557 = Select(t=w919, s=w908, f=u16 0) -> (s? t:f=w910:u16)
      n558 = Select(t=w917, s=w908, f=w920) -> (s? t:f=w909:u16)
      n559 = Replace Array Subset(array=w944, new element #1=w935, index #1=w932, new element #2=w934, index #2=w933, new element #3=w922, index #3=w924, new element #4=w921, index #4=w923, new element #5=w910, index #5=w912, new element #6=w909, index #6=w911) -> (w943:u16[])
    }
    frame 29 {
      # "Laser"
      # "Tcycle"
      # "count"
      # "Audio_R"
      # "Tcycle"
      # "count"
      # "Audio_L"
      # "Tcycle"
      # "count"
      # "Solenoid__L"
      # "Tcycle"
      # "count"
      n560 = call "myRIO_BRig_RT_dataMTrig_Solenoid_c__L.vi"() -> ("output_Solenoid_c__L"=w948:i32)  [unwired: 11 in]
      n561 = call "myRIO_BRig_RT_dataMTrig_Solenoid_Tcycle__L.vi"() -> ("output_Solenoid_Tcycle__L"=w951:i32)  [unwired: 11 in]
      n562 = call "myRIO_BRig_RT_dataMTrig_Audio_c__L.vi"() -> ("output_Audio_c__L"=w979:i32)  [unwired: 11 in]
      n563 = call "myRIO_BRig_RT_dataMTrig_Audio_Tcycle__L.vi"() -> ("output_Audio_Tcycle__L"=w985:i32)  [unwired: 11 in]
      n564 = call "myRIO_BRig_RT_dataMTrig_Audio_c__R.vi"() -> ("output_Audio_c__R"=w971:i32)  [unwired: 11 in]
      n565 = call "myRIO_BRig_RT_dataMTrig_Audio_Tcycle__R.vi"() -> ("output_Audio_Tcycle__R"=w972:i32)  [unwired: 11 in]
      n566 = call "myRIO_BRig_RT_dataMTrig_Laser_c.vi"() -> ("output_Laser_c"=w959:i32)  [unwired: 11 in]
      n567 = call "myRIO_BRig_RT_dataMTrig_Laser_Tcycle.vi"() -> ("output_Laser_Tcycle"=w962:i32)  [unwired: 11 in]
      n568 = Index Array(array=w992, index #1=w948, index #2=w951, index #3=w979, index #4=w985, index #5=w971, index #6=w972, index #7=w959, index #8=w962) -> (element #1=w950:u16, element #2=w949:u16, element #3=w984:u16, element #4=w983:u16, element #5=w974:u16, element #6=w973:u16, element #7=w961:u16, element #8=w960:u16)
      n569 = Add(x=w963, y=w950) -> (x+y=w994:u16)
      n570 = Add(x=w963, y=w984) -> (x+y=w988:u16)
      n571 = Add(x=w963, y=w974) -> (x+y=w977:u16)
      n572 = Add(x=w963, y=w961) -> (x+y=w966:u16)
      n573 = Less?(x=w994, y=w949) -> (x < y?=w952:bool)
      n574 = Less?(x=w988, y=w983) -> (x < y?=w953:bool)
      n575 = Less?(x=w977, y=w973) -> (x < y?=w954:bool)
      n576 = Less?(x=w966, y=w960) -> (x < y?=w955:bool)
      n577 = Decrement(x=w991) -> (x-1=w995:u16)
      n578 = Decrement(x=w986) -> (x-1=w989:u16)
      n579 = Decrement(x=w975) -> (x-1=w978:u16)
      n580 = Decrement(x=w964) -> (x-1=w967:u16)
      n581 = Select(t=w994, s=w952, f=u16 0) -> (s? t:f=w947:u16)
      n582 = Select(t=w991, s=w952, f=w995) -> (s? t:f=w945:u16)
      n583 = Select(t=w988, s=w953, f=u16 0) -> (s? t:f=w982:u16)
      n584 = Select(t=w986, s=w953, f=w989) -> (s? t:f=w981:u16)
      n585 = Select(t=w977, s=w954, f=u16 0) -> (s? t:f=w969:u16)
      n586 = Select(t=w975, s=w954, f=w978) -> (s? t:f=w968:u16)
      n587 = Select(t=w966, s=w955, f=u16 0) -> (s? t:f=w957:u16)
      n588 = Select(t=w964, s=w955, f=w967) -> (s? t:f=w956:u16)
      n589 = Replace Array Subset(array=w992, new element #1=w947, index #1=w948, new element #2=w945, index #2=w946, new element #3=w982, index #3=w979, new element #4=w981, index #4=w980, new element #5=w969, index #5=w971, new element #6=w968, index #6=w970, new element #7=w957, index #7=w959, new element #8=w956, index #8=w958) -> (w990:u16[])
    }
    frame 30 {
      # "Laser"
      # "Tcycle"
      # "count"
      # "Audio_R"
      # "Tcycle"
      # "count"
      # "Audio_L"
      # "Tcycle"
      # "count"
      # "Solenoid__R"
      # "Tcycle"
      # "count"
      n590 = call "myRIO_BRig_RT_dataMTrig_Solenoid_c__R.vi"() -> ("output_Solenoid_c__R"=w1038:i32)  [unwired: 11 in]
      n591 = call "myRIO_BRig_RT_dataMTrig_Solenoid_Tcycle__R.vi"() -> ("output_Solenoid_Tcycle__R"=w1041:i32)  [unwired: 11 in]
      n592 = call "myRIO_BRig_RT_dataMTrig_Audio_c__L.vi"() -> ("output_Audio_c__L"=w1023:i32)  [unwired: 11 in]
      n593 = call "myRIO_BRig_RT_dataMTrig_Audio_Tcycle__L.vi"() -> ("output_Audio_Tcycle__L"=w1029:i32)  [unwired: 11 in]
      n594 = call "myRIO_BRig_RT_dataMTrig_Audio_c__R.vi"() -> ("output_Audio_c__R"=w1015:i32)  [unwired: 11 in]
      n595 = call "myRIO_BRig_RT_dataMTrig_Audio_Tcycle__R.vi"() -> ("output_Audio_Tcycle__R"=w1016:i32)  [unwired: 11 in]
      n596 = call "myRIO_BRig_RT_dataMTrig_Laser_c.vi"() -> ("output_Laser_c"=w1003:i32)  [unwired: 11 in]
      n597 = call "myRIO_BRig_RT_dataMTrig_Laser_Tcycle.vi"() -> ("output_Laser_Tcycle"=w1006:i32)  [unwired: 11 in]
      n598 = Index Array(array=w1046, index #1=w1038, index #2=w1041, index #3=w1023, index #4=w1029, index #5=w1015, index #6=w1016, index #7=w1003, index #8=w1006) -> (element #1=w1040:u16, element #2=w1039:u16, element #3=w1028:u16, element #4=w1027:u16, element #5=w1018:u16, element #6=w1017:u16, element #7=w1005:u16, element #8=w1004:u16)
      n599 = Add(x=w1007, y=w1040) -> (x+y=w1044:u16)
      n600 = Add(x=w1007, y=w1028) -> (x+y=w1032:u16)
      n601 = Add(x=w1007, y=w1018) -> (x+y=w1021:u16)
      n602 = Add(x=w1007, y=w1005) -> (x+y=w1010:u16)
      n603 = Less?(x=w1044, y=w1039) -> (x < y?=w996:bool)
      n604 = Less?(x=w1032, y=w1027) -> (x < y?=w997:bool)
      n605 = Less?(x=w1021, y=w1017) -> (x < y?=w998:bool)
      n606 = Less?(x=w1010, y=w1004) -> (x < y?=w999:bool)
      n607 = Decrement(x=w1042) -> (x-1=w1045:u16)
      n608 = Decrement(x=w1030) -> (x-1=w1033:u16)
      n609 = Decrement(x=w1019) -> (x-1=w1022:u16)
      n610 = Decrement(x=w1008) -> (x-1=w1011:u16)
      n611 = Select(t=w1044, s=w996, f=u16 0) -> (s? t:f=w1037:u16)
      n612 = Select(t=w1042, s=w996, f=w1045) -> (s? t:f=w1035:u16)
      n613 = Select(t=w1032, s=w997, f=u16 0) -> (s? t:f=w1026:u16)
      n614 = Select(t=w1030, s=w997, f=w1033) -> (s? t:f=w1025:u16)
      n615 = Select(t=w1021, s=w998, f=u16 0) -> (s? t:f=w1013:u16)
      n616 = Select(t=w1019, s=w998, f=w1022) -> (s? t:f=w1012:u16)
      n617 = Select(t=w1010, s=w999, f=u16 0) -> (s? t:f=w1001:u16)
      n618 = Select(t=w1008, s=w999, f=w1011) -> (s? t:f=w1000:u16)
      n619 = Replace Array Subset(array=w1046, new element #1=w1037, index #1=w1038, new element #2=w1035, index #2=w1036, new element #3=w1026, index #3=w1023, new element #4=w1025, index #4=w1024, new element #5=w1013, index #5=w1015, new element #6=w1012, index #6=w1014, new element #7=w1001, index #7=w1003, new element #8=w1000, index #8=w1002) -> (w1034:u16[])
    }
    frame 31 {
      # "Laser"
      # "Tcycle"
      # "count"
      # "Audio_R"
      # "Tcycle"
      # "count"
      # "Audio_L"
      # "Tcycle"
      # "count"
      # "Solenoid__R"
      # "Tcycle"
      # "count"
      # "Solenoid__L"
      # "Tcycle"
      # "count"
      n620 = call "myRIO_BRig_RT_dataMTrig_Solenoid_c__L.vi"() -> ("output_Solenoid_c__L"=w1098:i32)  [unwired: 11 in]
      n621 = call "myRIO_BRig_RT_dataMTrig_Solenoid_Tcycle__L.vi"() -> ("output_Solenoid_Tcycle__L"=w1109:i32)  [unwired: 11 in]
      n622 = call "myRIO_BRig_RT_dataMTrig_Solenoid_c__R.vi"() -> ("output_Solenoid_c__R"=w1090:i32)  [unwired: 11 in]
      n623 = call "myRIO_BRig_RT_dataMTrig_Solenoid_Tcycle__R.vi"() -> ("output_Solenoid_Tcycle__R"=w1093:i32)  [unwired: 11 in]
      n624 = call "myRIO_BRig_RT_dataMTrig_Audio_c__L.vi"() -> ("output_Audio_c__L"=w1075:i32)  [unwired: 11 in]
      n625 = call "myRIO_BRig_RT_dataMTrig_Audio_Tcycle__L.vi"() -> ("output_Audio_Tcycle__L"=w1081:i32)  [unwired: 11 in]
      n626 = call "myRIO_BRig_RT_dataMTrig_Audio_c__R.vi"() -> ("output_Audio_c__R"=w1067:i32)  [unwired: 11 in]
      n627 = call "myRIO_BRig_RT_dataMTrig_Audio_Tcycle__R.vi"() -> ("output_Audio_Tcycle__R"=w1068:i32)  [unwired: 11 in]
      n628 = call "myRIO_BRig_RT_dataMTrig_Laser_c.vi"() -> ("output_Laser_c"=w1055:i32)  [unwired: 11 in]
      n629 = call "myRIO_BRig_RT_dataMTrig_Laser_Tcycle.vi"() -> ("output_Laser_Tcycle"=w1058:i32)  [unwired: 11 in]
      n630 = Index Array(array=w1103, index #1=w1098, index #2=w1109, index #3=w1090, index #4=w1093, index #5=w1075, index #6=w1081, index #7=w1067, index #8=w1068, index #9=w1055, index #10=w1058) -> (element #1=w1108:u16, element #2=w1107:u16, element #3=w1092:u16, element #4=w1091:u16, element #5=w1080:u16, element #6=w1079:u16, element #7=w1070:u16, element #8=w1069:u16, element #9=w1057:u16, element #10=w1056:u16)
      n631 = Add(x=w1059, y=w1108) -> (x+y=w1105:u16)
      n632 = Add(x=w1059, y=w1092) -> (x+y=w1096:u16)
      n633 = Add(x=w1059, y=w1080) -> (x+y=w1084:u16)
      n634 = Add(x=w1059, y=w1070) -> (x+y=w1073:u16)
      n635 = Add(x=w1059, y=w1057) -> (x+y=w1062:u16)
      n636 = Less?(x=w1105, y=w1107) -> (x < y?=w1047:bool)
      n637 = Less?(x=w1096, y=w1091) -> (x < y?=w1048:bool)
      n638 = Less?(x=w1084, y=w1079) -> (x < y?=w1049:bool)
      n639 = Less?(x=w1073, y=w1069) -> (x < y?=w1050:bool)
      n640 = Less?(x=w1062, y=w1056) -> (x < y?=w1051:bool)
      n641 = Decrement(x=w1100) -> (x-1=w1106:u16)
      n642 = Decrement(x=w1094) -> (x-1=w1097:u16)
      n643 = Decrement(x=w1082) -> (x-1=w1085:u16)
      n644 = Decrement(x=w1071) -> (x-1=w1074:u16)
      n645 = Decrement(x=w1060) -> (x-1=w1063:u16)
      n646 = Select(t=w1105, s=w1047, f=u16 0) -> (s? t:f=w1101:u16)
      n647 = Select(t=w1100, s=w1047, f=w1106) -> (s? t:f=w1102:u16)
      n648 = Select(t=w1096, s=w1048, f=u16 0) -> (s? t:f=w1089:u16)
      n649 = Select(t=w1094, s=w1048, f=w1097) -> (s? t:f=w1087:u16)
      n650 = Select(t=w1084, s=w1049, f=u16 0) -> (s? t:f=w1078:u16)
      n651 = Select(t=w1082, s=w1049, f=w1085) -> (s? t:f=w1077:u16)
      n652 = Select(t=w1073, s=w1050, f=u16 0) -> (s? t:f=w1065:u16)
      n653 = Select(t=w1071, s=w1050, f=w1074) -> (s? t:f=w1064:u16)
      n654 = Select(t=w1062, s=w1051, f=u16 0) -> (s? t:f=w1053:u16)
      n655 = Select(t=w1060, s=w1051, f=w1063) -> (s? t:f=w1052:u16)
      n656 = Replace Array Subset(array=w1103, new element #1=w1101, index #1=w1098, new element #2=w1102, index #2=w1099, new element #3=w1089, index #3=w1090, new element #4=w1087, index #4=w1088, new element #5=w1078, index #5=w1075, new element #6=w1077, index #6=w1076, new element #7=w1065, index #7=w1067, new element #8=w1064, index #8=w1066, new element #9=w1053, index #9=w1055, new element #10=w1052, index #10=w1054) -> (w1086:u16[])
    }
  }
  "output_dataMTrig" <- w9
  "output_Solenoid_L" <- w5
  "output_Solenoid_R" <- w4
  "output_Audio_L" <- w3
  "output_Audio_R" <- w2
  "output_Laser" <- w1
